vi "Lockin-4461 -Patrick -State -IV.vi"(11 "Channels: AO":T8={"AO amp (V)"=[1.0, 0.0, 0.0, 0.0, 0.0, 0.0, 0.0, 0.0], "AO DC (V)"=[0.0, 0.0, 0.0, 0.0, 0.0, 0.0, 0.0, 0.0], "AO f (Hz)"=[0.4, 0.4, 0.4, 0.4, 0.4, 0.4, 0.4, 0.4], "AO phi (deg)"=[0.0, 0.0, 0.0, 0.0, 0.0, 0.0, 0.0, 0.0], "function"=[enum."Triangle Wave", enum."Sine Wave", enum."Sine Wave", enum."Sine Wave", enum."Sine Wave", enum."Sine Wave", enum."Sine Wave", enum."Sine Wave"]} {"AO f (Hz)" min=0.001 max=1000.0; "AO DC (V)" format="%#_6p"; "AO amp (V)" format="%#_6p"}) -> ()   [LabVIEW 2013]
uses:
  <vilib>/Analysis/4window.llb/windowTd.ctl
  <vilib>/measure/maspectr.llb/Power Spectrum and PSD Export Mode.ctl
  <vilib>/Utility/error.llb/DialogType.ctl
  <vilib>/Analysis/baseanly.llb/Mean (DBL).vi
  <vilib>/Analysis/2dsp.llb/Decimate (single shot).vi
  <vilib>/Analysis/2dsp.llb/Decimate (single shot, DBL).vi
  <userlib>/_OpenG.lib/array/array.llb/Empty 1D Array (Variant)__ogtk.vi
  <userlib>/_OpenG.lib/array/array.llb/Empty 1D Array (DBL)__ogtk.vi
  <vilib>/measure/maspectr.llb/FFT Power Spectrum and PSD for N Chan.vi
  <vilib>/Waveform/WDTOps.llb/WDT Waveform to XY Pairs DBL.vi
  <vilib>/measure/NI_MAPro.lvlib
  <vilib>/Analysis/NI_AALBase.lvlib
  <vilib>/platform/TimedLoop/XDataNode/XDataNode.xnode
  <vilib>/Platform/TimedLoop/XDataNode/nitl_modes.ctl
  <vilib>/Platform/TimedLoop/XDataNode/XDNodeRunTimeDep.lvlib
  <vilib>/Platform/TimedLoop/XDataNode/wakeup.ctl
  <vilib>/Platform/TimedLoop/XDataNode/timing_clust.ctl
  <vilib>/Analysis/NI_AALPro.lvlib
panel:
  in  "save interval (s)":dbl=300.0
  out "save time":timestamp
  out "Error":bool
  out "Results\n(X, Y, R, Theta, mean)":dbl[][](array[numeric])=[[0.8094339767492822, -0.005512419987470585, 0.8094527469162581, -0.3901905858084899, -6.0129843950271606e-05], [-1.260821172105524e-07, 2.7497299313388556e-07, 3.0250098716087416e-07, 114.63266099744331, 0.0001555195415019989], [7.489149035008232e-07, 4.842270951726359e-07, 8.918236442172725e-07, 32.88556061807632, 8.126195073127747e-05], [-1.8506084817561703e-07, 1.6463385705296426e-07, 2.476930043735887e-07, 138.34306439782742, 0.0027563392603397368], [-4.6280871026111895e-07, 4.8028636431280393e-08, 4.652941566482524e-07, 174.07525665627907, 0.002910439200401306], [-4.1354357574928766e-07, 2.831131466682128e-07, 5.011699740206747e-07, 145.60434384741927, 0.0028921316146850585], [0.8094339767492822, -0.005512419987470585, 0.8094527469162581, -0.3901905858084899, 0.0], [-1.260821172105524e-07, 2.7497299313388556e-07, 3.0250098716087416e-07, 114.63266099744331, 0.0], [7.489149035008232e-07, 4.842270951726359e-07, 8.918236442172725e-07, 32.88556061807632, 0.0], [-1.8506084817561703e-07, 1.6463385705296426e-07, 2.476930043735887e-07, 138.34306439782742, 0.0], [-4.6280871026111895e-07, 4.8028636431280393e-08, 4.652941566482524e-07, 174.07525665627907, 0.0], [-4.1354357574928766e-07, 2.831131466682128e-07, 5.011699740206747e-07, 145.60434384741927, 0.0]] format="%#_3p"
  out "current time":timestamp=timestamp(3547741041.3268714 s since 1904-01-01)
  in  "Channel":dbl min=0.0 max=7.0 step=1.0
  in  "Display":enum16{"X and Y", "R and Theta"}(ring)
  out "Y or Theta":dbl=-0.005512419987470585 caption="Y or Theta: Current (A) or Voltage (V)" format="%.3p"
  out "X or R":dbl=0.8094339767492822 caption="X or R: Current (A) or Voltage (V)" format="%#.3p"
  in  "Save Data":bool
  in  "RESET":bool
  in  "EXIT":bool
  in  "path":path=path "C:/Data/lockin"
  in  "Notes":string
  in  "mean":dbl[](array[numeric])=[-6.0129843950271606e-05, 0.0001555195415019989, 8.126195073127747e-05, 0.0027563392603397368, 0.002910439200401306, 0.0028921316146850585]
  in  "Tab Control 2":T1(tab)
  in  "Output signals?":bool
  out "Signals Graph":waveform(dbl)[](graph)=[{"t0"=timestamp(3547741038.80007 s since 1904-01-01), "dt"=0.0002499999997785377, "Y"=array[10000 elements], "attributes"=variant("NI_ChannelName"=variant(string "PXI1Slot2/ai0"), "NI_UnitDescription"=variant(string "Volts"))}, {"t0"=timestamp(3547741038.80007 s since 1904-01-01), "dt"=0.0002499999997785377, "Y"=array[10000 elements], "attributes"=variant("NI_ChannelName"=variant(string "PXI1Slot2/ai1"), "NI_UnitDescription"=variant(string "Volts"))}, {"t0"=timestamp(3547741038.800245 s since 1904-01-01), "dt"=0.0002499999997785377, "Y"=array[10000 elements], "attributes"=variant("NI_ChannelName"=variant(string "PXI1Slot3/ai0"), "NI_UnitDescription"=variant(string "Volts"))}, {"t0"=timestamp(3547741038.800245 s since 1904-01-01), "dt"=0.0002499999997785377, "Y"=array[10000 elements], "attributes"=variant("NI_ChannelName"=variant(string "PXI1Slot3/ai1"), "NI_UnitDescription"=variant(string "Volts"))}, {"t0"=timestamp(3547741038.800295 s since 1904-01-01), "dt"=0.0002499999997785377, "Y"=array[10000 elements], "attributes"=variant("NI_ChannelName"=variant(string "PXI1Slot5/ai0"), "NI_UnitDescription"=variant(string "Volts"))}, {"t0"=timestamp(3547741038.800295 s since 1904-01-01), "dt"=0.0002499999997785377, "Y"=array[10000 elements], "attributes"=variant("NI_ChannelName"=variant(string "PXI1Slot5/ai1"), "NI_UnitDescription"=variant(string "Volts"))}]
  out "Reference Graph":waveform(dbl)[](graph)=[{"t0"=timestamp(3547741038.7997265 s since 1904-01-01), "dt"=0.00025, "Y"=array[10000 elements]}, {"t0"=timestamp(3547741038.7997265 s since 1904-01-01), "dt"=0.00025, "Y"=array[10000 elements]}, {"t0"=timestamp(3547741038.7997265 s since 1904-01-01), "dt"=0.00025, "Y"=array[10000 elements]}, {"t0"=timestamp(3547741038.7997265 s since 1904-01-01), "dt"=0.00025, "Y"=array[10000 elements]}, {"t0"=timestamp(3547741038.7997265 s since 1904-01-01), "dt"=0.00025, "Y"=array[10000 elements]}, {"t0"=timestamp(3547741038.7997265 s since 1904-01-01), "dt"=0.00025, "Y"=array[10000 elements]}, {"t0"=timestamp(3547741038.7997265 s since 1904-01-01), "dt"=0.00025, "Y"=array[10000 elements]}, {"t0"=timestamp(3547741038.7997265 s since 1904-01-01), "dt"=0.00025, "Y"=array[10000 elements]}]
  in  "decimate graph":i32=10
  in  "Display n?":bool
  out "Gauge":dbl(knob)=21.0 scale=0.0..60.0
  out "Display X (or R)":waveform(dbl)[](graph)=[{"t0"=timestamp(3547741038.80007 s since 1904-01-01), "dt"=1.0, "Y"=[0.8094339767492822]}, {"t0"=timestamp(3547741038.80007 s since 1904-01-01), "dt"=1.0, "Y"=[-1.260821172105524e-07]}, {"t0"=timestamp(3547741038.80007 s since 1904-01-01), "dt"=1.0, "Y"=[7.489149035008232e-07]}, {"t0"=timestamp(3547741038.80007 s since 1904-01-01), "dt"=1.0, "Y"=[-1.8506084817561703e-07]}, {"t0"=timestamp(3547741038.80007 s since 1904-01-01), "dt"=1.0, "Y"=[-4.6280871026111895e-07]}, {"t0"=timestamp(3547741038.80007 s since 1904-01-01), "dt"=1.0, "Y"=[-4.1354357574928766e-07]}, {"t0"=timestamp(3547741038.80007 s since 1904-01-01), "dt"=1.0, "Y"=[0.8094339767492822]}, {"t0"=timestamp(3547741038.80007 s since 1904-01-01), "dt"=1.0, "Y"=[-1.260821172105524e-07]}, {"t0"=timestamp(3547741038.80007 s since 1904-01-01), "dt"=1.0, "Y"=[7.489149035008232e-07]}, {"t0"=timestamp(3547741038.80007 s since 1904-01-01), "dt"=1.0, "Y"=[-1.8506084817561703e-07]}, {"t0"=timestamp(3547741038.80007 s since 1904-01-01), "dt"=1.0, "Y"=[-4.6280871026111895e-07]}, {"t0"=timestamp(3547741038.80007 s since 1904-01-01), "dt"=1.0, "Y"=[-4.1354357574928766e-07]}]
  out "Display Y (or Theta)":waveform(dbl)[](graph)=[{"t0"=timestamp(3547741038.80007 s since 1904-01-01), "dt"=1.0, "Y"=[-0.005512419987470585]}, {"t0"=timestamp(3547741038.80007 s since 1904-01-01), "dt"=1.0, "Y"=[2.7497299313388556e-07]}, {"t0"=timestamp(3547741038.80007 s since 1904-01-01), "dt"=1.0, "Y"=[4.842270951726359e-07]}, {"t0"=timestamp(3547741038.80007 s since 1904-01-01), "dt"=1.0, "Y"=[1.6463385705296426e-07]}, {"t0"=timestamp(3547741038.80007 s since 1904-01-01), "dt"=1.0, "Y"=[4.8028636431280393e-08]}, {"t0"=timestamp(3547741038.80007 s since 1904-01-01), "dt"=1.0, "Y"=[2.831131466682128e-07]}, {"t0"=timestamp(3547741038.80007 s since 1904-01-01), "dt"=1.0, "Y"=[-0.005512419987470585]}, {"t0"=timestamp(3547741038.80007 s since 1904-01-01), "dt"=1.0, "Y"=[2.7497299313388556e-07]}, {"t0"=timestamp(3547741038.80007 s since 1904-01-01), "dt"=1.0, "Y"=[4.842270951726359e-07]}, {"t0"=timestamp(3547741038.80007 s since 1904-01-01), "dt"=1.0, "Y"=[1.6463385705296426e-07]}, {"t0"=timestamp(3547741038.80007 s since 1904-01-01), "dt"=1.0, "Y"=[4.8028636431280393e-08]}, {"t0"=timestamp(3547741038.80007 s since 1904-01-01), "dt"=1.0, "Y"=[2.831131466682128e-07]}]
  out "XY Graph":cluster{dbl[], dbl[]}[](graph)=[{[0.0, 0.8094339767492822], [0.0, -0.005512419987470585]}, {[0.0, -1.260821172105524e-07], [0.0, 2.7497299313388556e-07]}, {[0.0, 7.489149035008232e-07], [0.0, 4.842270951726359e-07]}, {[0.0, -1.8506084817561703e-07], [0.0, 1.6463385705296426e-07]}, {[0.0, -4.6280871026111895e-07], [0.0, 4.8028636431280393e-08]}, {[0.0, -4.1354357574928766e-07], [0.0, 2.831131466682128e-07]}, {[0.0, 0.8094339767492822], [0.0, -0.005512419987470585]}, {[0.0, -1.260821172105524e-07], [0.0, 2.7497299313388556e-07]}, {[0.0, 7.489149035008232e-07], [0.0, 4.842270951726359e-07]}, {[0.0, -1.8506084817561703e-07], [0.0, 1.6463385705296426e-07]}, {[0.0, -4.6280871026111895e-07], [0.0, 4.8028636431280393e-08]}, {[0.0, -4.1354357574928766e-07], [0.0, 2.831131466682128e-07]}]
  out "PS Chart":dbl[][](graph)=[[-1411.497616925462, -1404.3790029743438, -1413.0961920610762, -1418.6418791322994, -1413.136726104145, -1413.4151534226191, -1417.9246313001065, -1424.6072395567076]]
  out "PS dB":cluster{"f0":dbl, "df":dbl, "magnitude":dbl[]}[](graph)
  in  "window":T2=1 items=["Rectangle"=0, "Hanning"=1, "Hamming"=2, "Blackman-Harris"=3, "Exact Blackman"=4, "Blackman"=5, "Flat Top"=6, "4 Term B-Harris "=7, "7 Term B-Harris"=8, "Low Sidelobe"=9, "Blackman Nuttall"=11, "Triangle"=30, "Bartlett-Hanning"=31, "Bohman"=32, "Parzen"=33, "Welch"=34, "Kaiser"=60, "Dolph-Chebyshev"=61, "Gaussian"=62]
  in  "averaging parameters":T3={"averaging mode"=enum."RMS averaging", "weighting mode"=enum."Exponential", "number of averages"=10} {"number of averages" min=1}
  in  "restart averaging (F)":bool
  in  "export mode":T4 items=["Power Spectrum", "Power Spectral Density"]
  in  "window parameter":dbl=nan
  out "averages\ncompleted":dbl=8319.0
  out "averaging done":bool=TRUE
  in  "Tab Control":T5(tab)=enum."AO/Lockin Setup"
  in  "decimating factor":i32=1
  in  "AI Buffer Size (S)":i32=100
  out "dt":dbl=2.5e-05 format="%#_6p"
  in  "AO Configuration":T6(array[cluster])=[{"Output physical channels"="PXI1Slot2/ao0:1", "AO. Max"=1.0, "AO.Min"=-1.0}, {"Output physical channels"="PXI1Slot3/ao0:1", "AO. Max"=1.0, "AO.Min"=-1.0}, {"Output physical channels"="PXI1Slot5/ao0:1", "AO. Max"=1.0, "AO.Min"=-1.0}]
  in  "AI Configuration":T7(array[cluster])=[{"AI.Coupling"=10050, "AI.Max"=1.0, "AI.Min"=-1.0, "Input physical channels"="PXI1Slot2/ai0:1"}, {"AI.Coupling"=10050, "AI.Max"=1.0, "AI.Min"=-1.0, "Input physical channels"="PXI1Slot3/ai0:1"}, {"AI.Coupling"=10050, "AI.Max"=1.0, "AI.Min"=-1.0, "Input physical channels"="PXI1Slot5/ai0:1"}] {"AI.Coupling" items=["AC"=10045, "DC"=10050, "GND"=10066]}
  out "error":errorcluster
  in  "IV curves?":bool=TRUE
  in  "measure offset":bool
  in  "reset signal":bool
  in  "all  f same?":bool
  in  "reset REF phi to zero":bool
  in  "zero offset":bool
  in  "LP cutoff (Hz)":dbl=10.0
  in  "LP prefilter":bool
  in  "60 Hz prefilter":bool
  in  "Wait on Trigger":bool
  in  "Remote Mode":bool
  in  "Channels: Lockin":T9={"REF f (Hz)"=[0.4, 0.4], "REF phi (deg)"=[0.0, 0.0]} {"REF phi (deg)" format="%#_3g"}
  in  "simulate?":bool
  in  "order":i32=2
  in  "TC (s)":dbl=0.01 format="%#_6p"
  out "filter fC (Hz)":dbl=0.3183098861837907
  in  "autophase?\n(experimental)":bool
  in  "P":dbl=0.5 format="%.2f"
  in  "I":dbl=0.6 format="%.2f"
  in  "D":dbl=0.019999999999999997 format="%.2f"
  out "time since trigger":dbl
  in  "auto block size":bool=TRUE
  in  "x":dbl=100000.0 format="%#_13g"
  in  "sampling info":cluster{"Fs":i32, "#s":i32}={"Fs"=40000, "#s"=100000}
  in  "offsets":dbl[](array[numeric])=[0.0, 0.0, 0.0, 0.0, 0.0, 0.0, 0.0, 0.0] format="%#.2p"
  in  "Gain":dbl[](array[numeric])=[1.0, 1.0, 1.0, 1.0, 1.0, 1.0, 1.0, 1.0]
  out "phase log":dbl[](array[numeric])=[12.0, 12.0, 12.0, 12.0, 12.0, 12.0, 12.0, 12.0] format="%.1f"
  # "´"
  # "Multichannel Lockin v2016/06/02 IV"
  # "this is disabled!"
  # "plot 0    = AI0 f0\nplot 1    = Ai1 f0\n...\nplot N-1  = AIN f0\n\nplot N    = AI0 f1\nplot N+1  = AI1 f1\n..."
  # "sampling"
  # "prefilters"
  # "Make fs x*f0"
  # "lockin filter"
  # "autophase"
  # "0"
  # "1"
  # "2"
  # "3"
  # "4"
  # "5"
  # "6"
  # "7"
  # "Random Thoughts\n1. change the path in the yellow box below where you want to save the signal traces for diagnostics\n(G:\\ on CustardPie, H:\\ on WindySea)\n2. Change the AI and AO limits on the DAQ Settings tab\n\nPlease email p.irvin@levylab.org with questions or suggestions. Thanks."
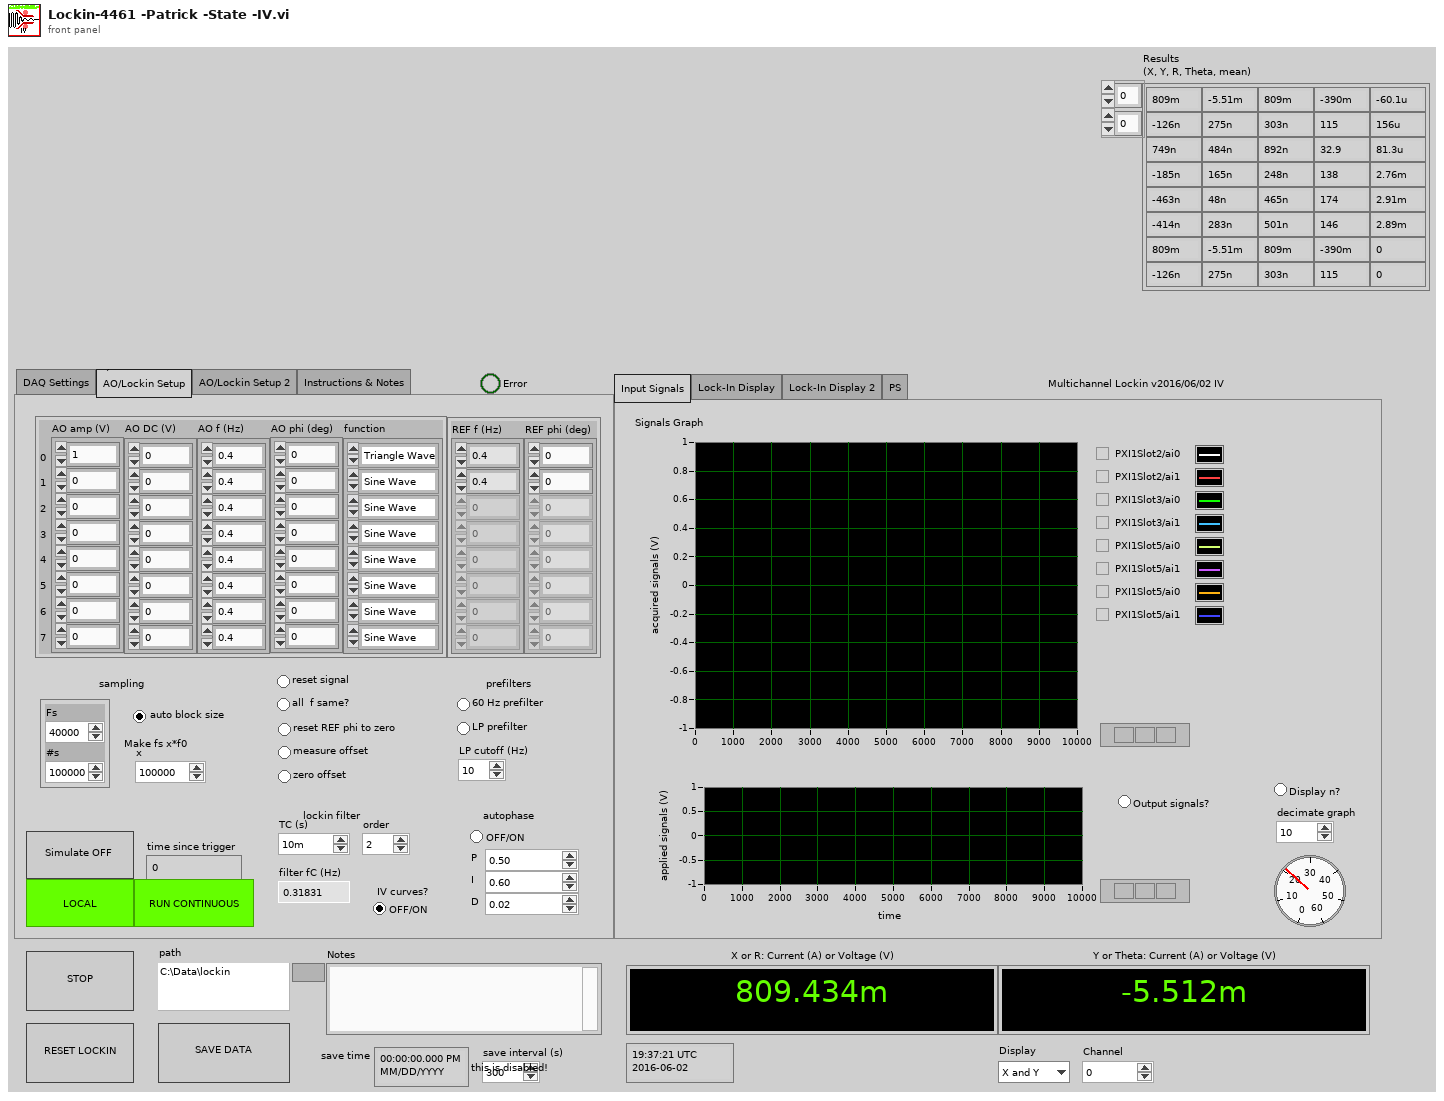
[diagram p1: front panel]
types:
  T1 = enum32{"Input Signals", "Lock-In Display", "Lock-In Display 2", "PS"}
  T2 = typedef "NI_AALPro.lvlib/windowTd.ctl" = u32
  T3 = cluster{"averaging mode":enum16{"No averaging", "Vector averaging", "RMS averaging", "Peak hold"}, "weighting mode":enum16{"Linear", "Exponential"}, "number of averages":u32}
  T4 = typedef "NI_MAPro.lvlib/Power Spectrum and PSD Export Mode.ctl" = u16
  T5 = enum32{"DAQ Settings", "AO/Lockin Setup", "AO/Lockin Setup 2", "Instructions & Notes"}
  T6 = cluster{"Output physical channels":tag, "AO. Max":dbl, "AO.Min":dbl}[]
  T7 = cluster{"AI.Coupling":i32, "AI.Max":dbl, "AI.Min":dbl, "Input physical channels":tag}[]
  T8 = cluster{"AO amp (V)":dbl[], "AO DC (V)":dbl[], "AO f (Hz)":dbl[], "AO phi (deg)":dbl[], "function":enum16{"Sine Wave", "Triangle Wave", "Square Wave", "Sawtooth Wave"}[]}
  T9 = cluster{"REF f (Hz)":dbl[], "REF phi (deg)":dbl[]}
  T10 = typedef "XDNodeRunTimeDep.lvlib/timing_clust.ctl" = cluster{"Expected End [f-1]":u64, "Actual End [f-1]":u64, "Finished Late? [f-1]":bool, "Expected End [i-1]":u64, "Actual End [i-1]":u64, "Finished Late? [i-1]":bool, "Expected Start [i]":u64, "Actual Start [i]":u64, "Expected Start [f]":u64, "Actual Start [f]":u64, "Source Name":string, "Structure Name":string, "Period":i64, "Deadline":i64, "Offset":i64, "Start":i64, "Priority":i32, "Timeout":i32, "Mode":T11, "Wakeup Reason":T12, "Error":errorcluster, "Source Type":string, "Secondary Source Type":string, "Global End Time":u64, "Global Start Time":u64, "Frame Duration":u64, "Iteration Duration":u64, "Assigned CPU":i32, "I/O Scan Engine Mode":u32}
  T11 = typedef "XDNodeRunTimeDep.lvlib/nitl_modes.ctl" = enum32{"No Change", "Process missed periods, maintain original phase", "Discard missed periods, maintain original phase", "Process missed periods, ignore original phase", "Discard missed periods, ignore original phase"}
  T12 = typedef "XDNodeRunTimeDep.lvlib/wakeup.ctl" = enum32{"Normal", "Aborted", "Asynchronous wakeup", "Timing source error", "Timed loop error", "Timeout"}
  T13 = enum32{"invalid app kind", "Development System", "Run Time System", "Student Edition", "Embedded LabVIEW", "Evaluation", "Custom"}
  T14 = enum32{"Invalid", "Standard", "Closed", "Hidden", "Minimized", "Maximized"}
  T15 = enum32{"Input Signals", "Lock-In Display", "Lock-In Display 2", "PS", "FFT"}
  T16 = cluster{"Core":cluster{"Current VI Reference":refnum<vi>, "Close Panel on Exit?":bool}, "Error":bool, "Your string data":string, "AI task":refnum<k21>[], "AO task":refnum<k21>[], "Input Signals":waveform(dbl)[], "Ouput Signals":waveform(dbl)[], "REF":waveform(dbl)[], "sampling info":cluster{"Fs":dbl, "#s":dbl}}
  T17 = typedef "DialogType.ctl" = u16
  T18 = cluster{"Current VI Reference":refnum<vi>, "Close Panel on Exit?":bool}
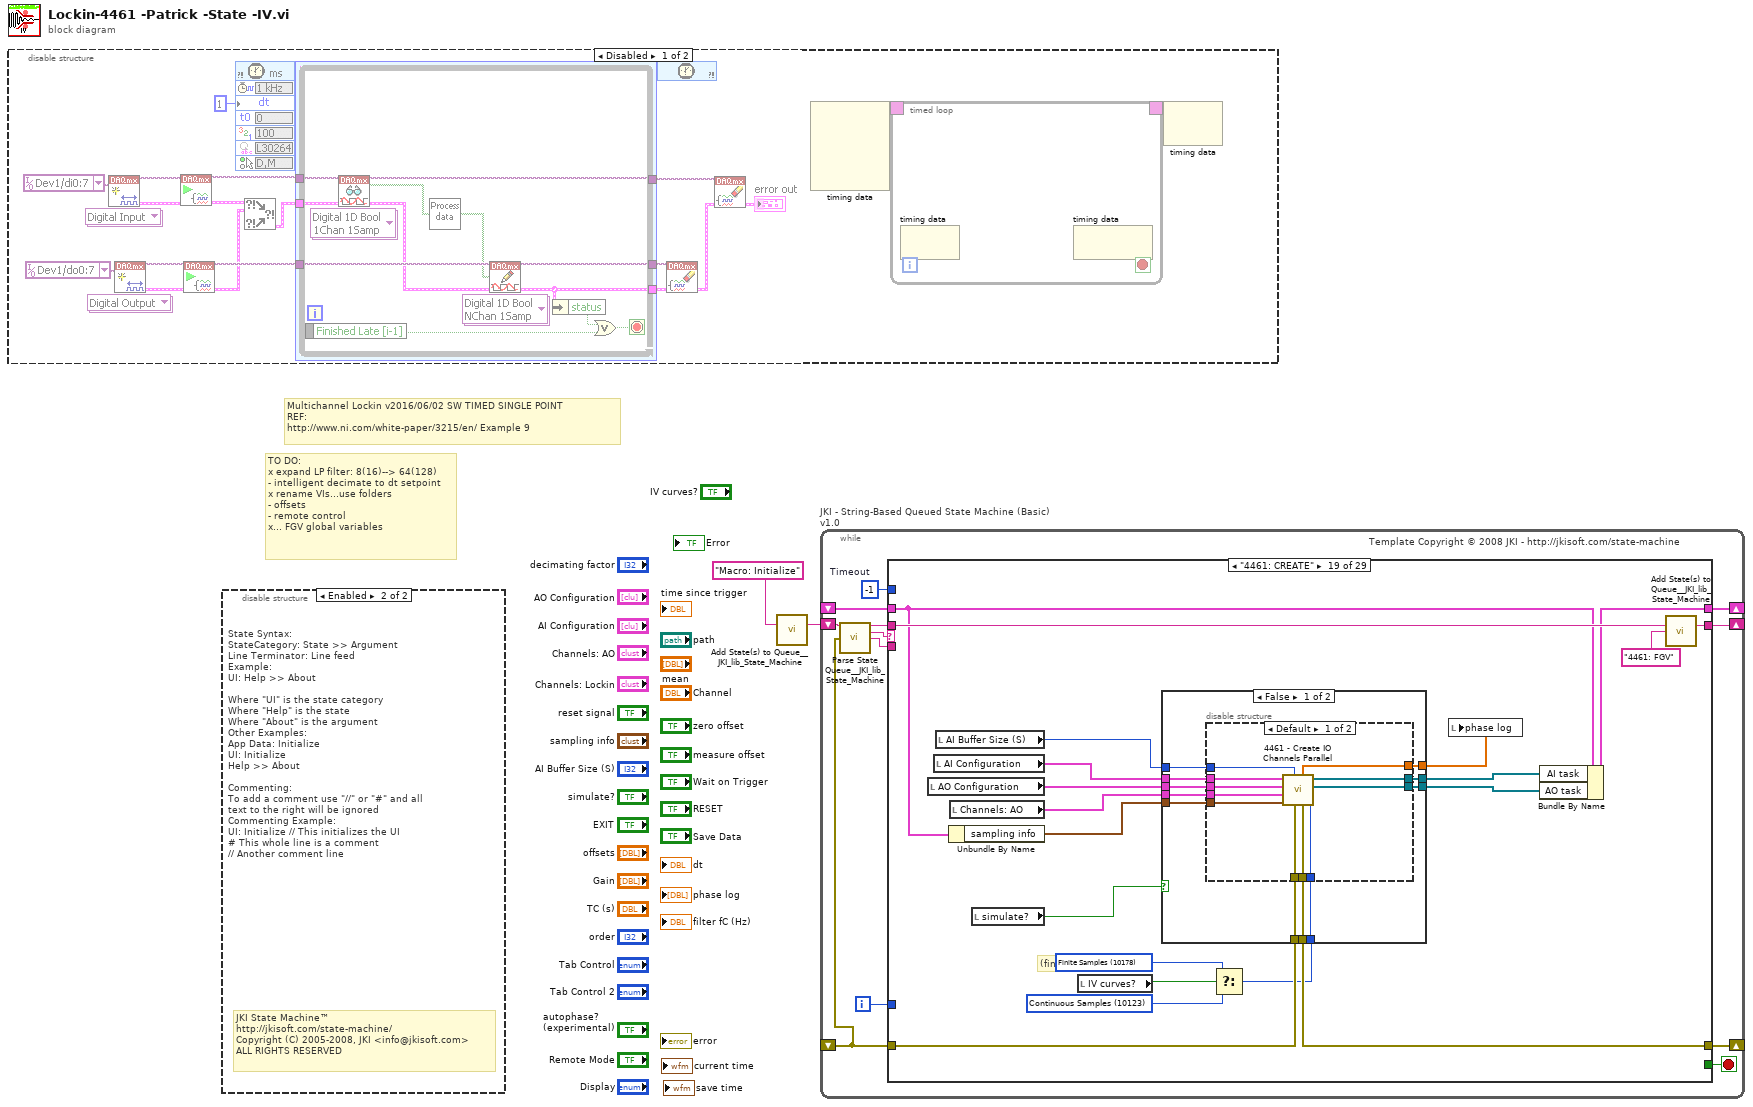
[diagram p0: block diagram]
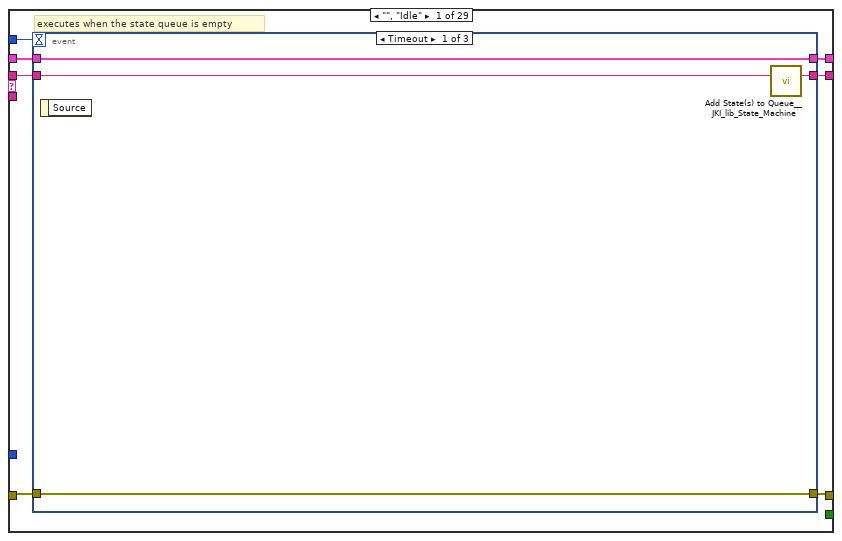
[diagram p4: hidden frame]
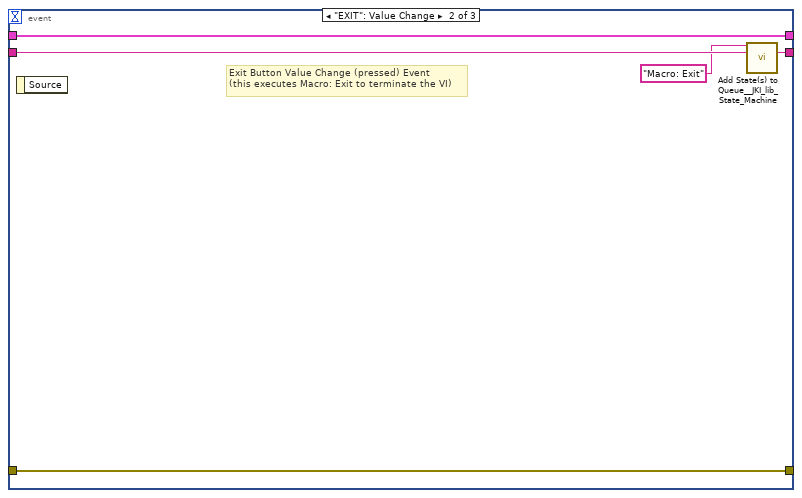
[diagram p5: hidden frame]
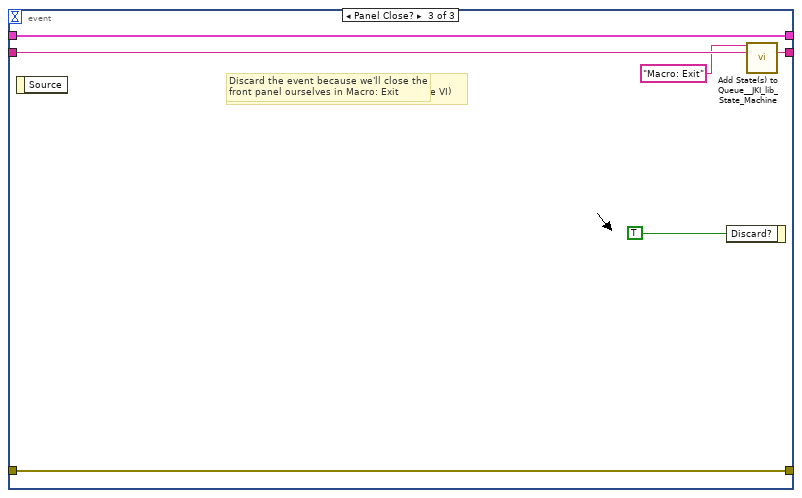
[diagram p6: hidden frame]
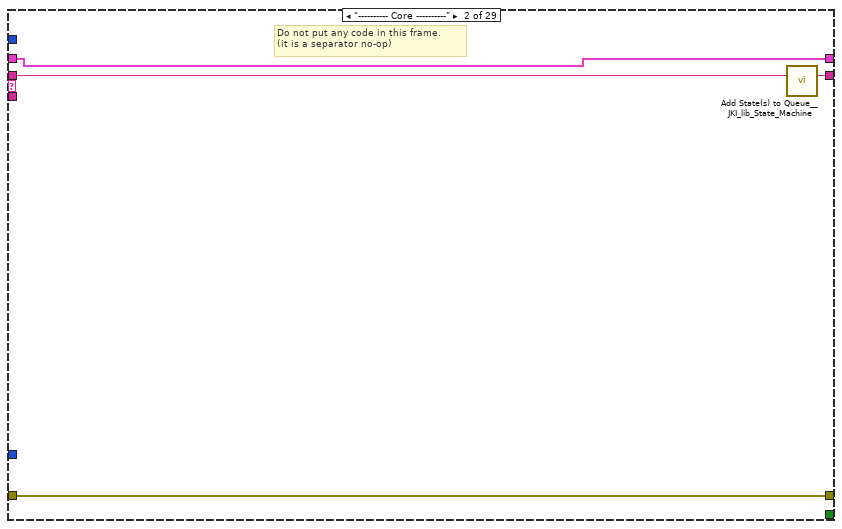
[diagram p7: hidden frame]
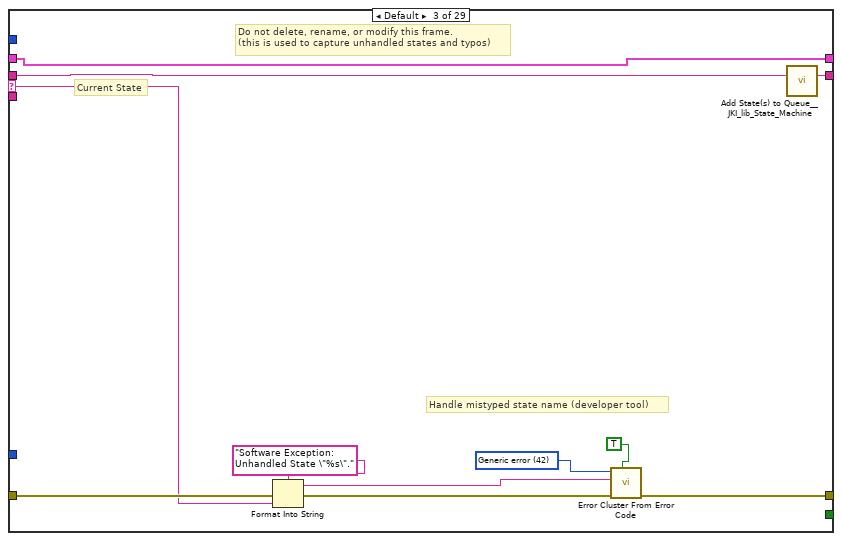
[diagram p8: hidden frame]
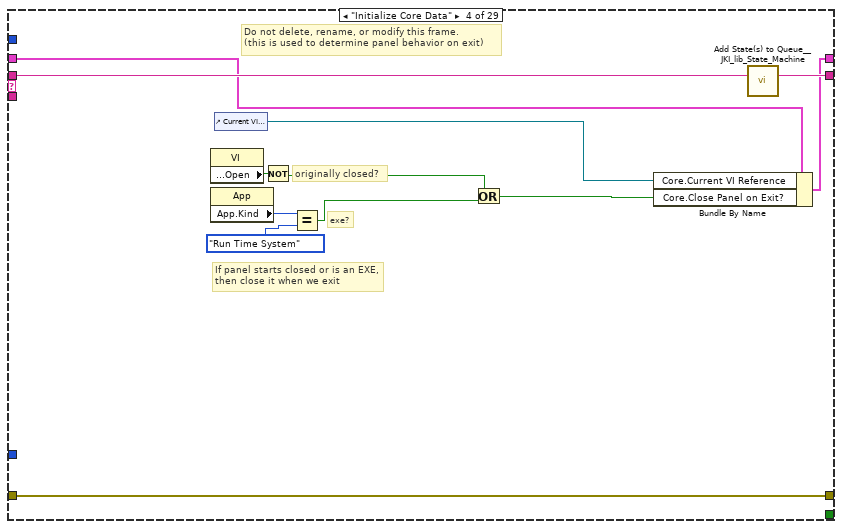
[diagram p9: hidden frame]
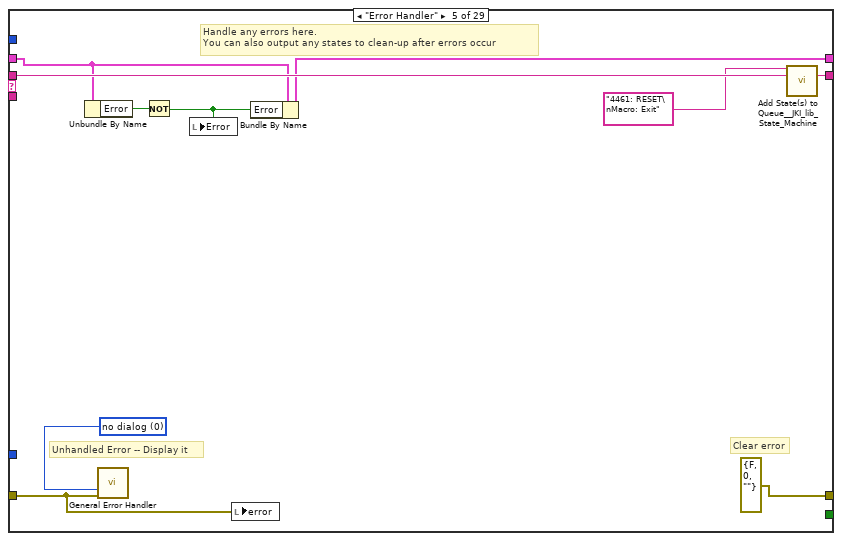
[diagram p10: hidden frame]
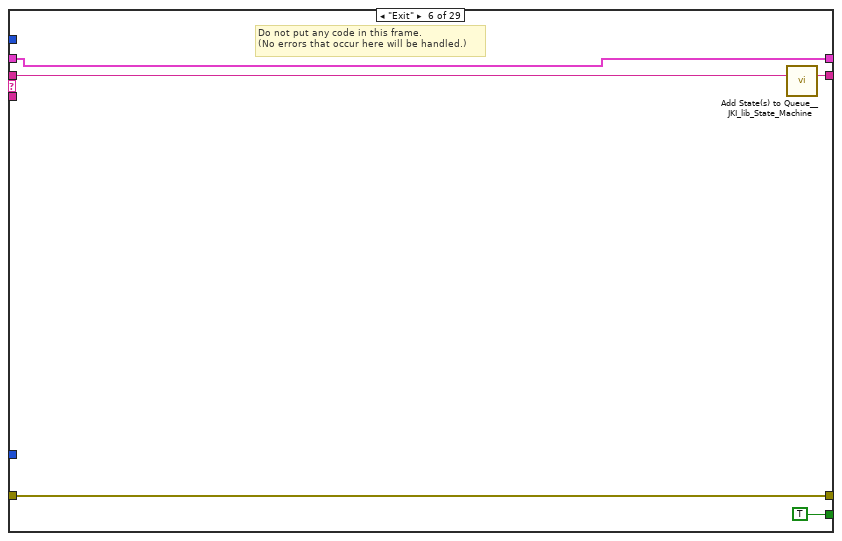
[diagram p11: hidden frame]
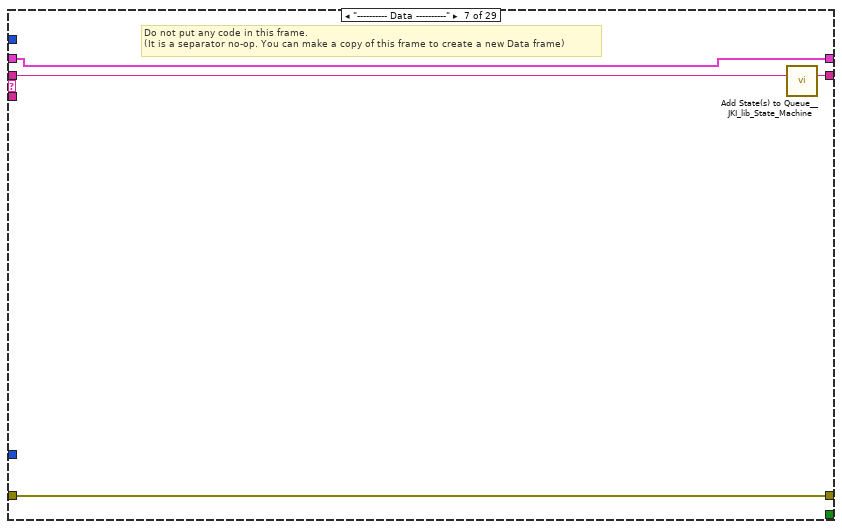
[diagram p12: hidden frame]
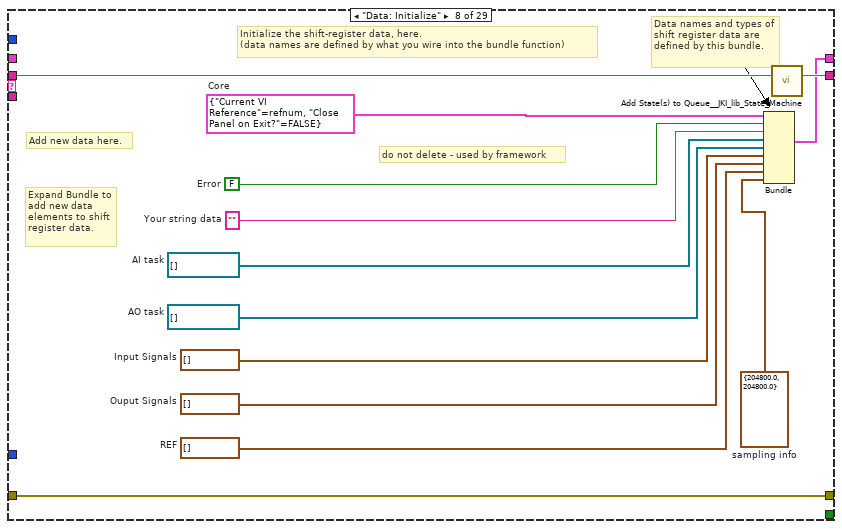
[diagram p13: hidden frame]
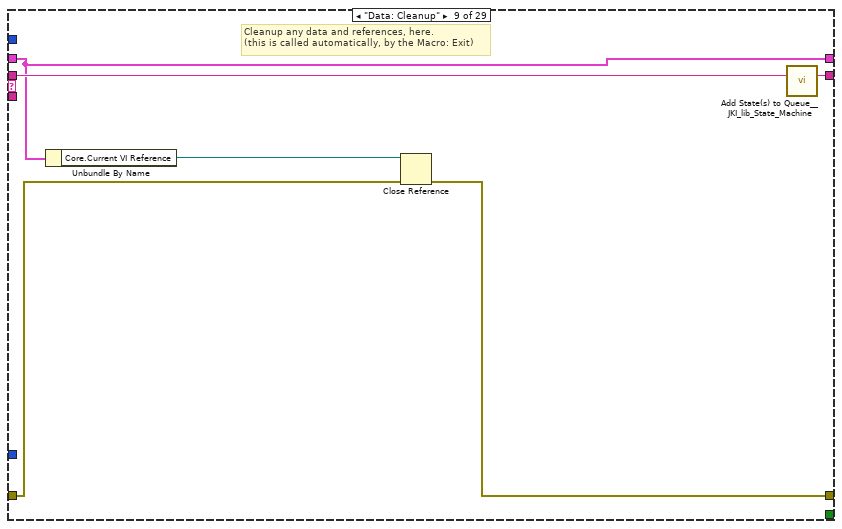
[diagram p14: hidden frame]
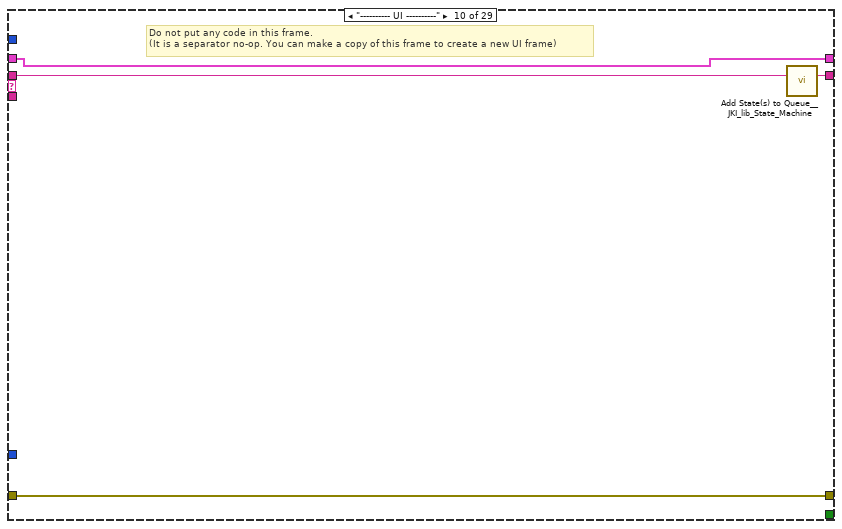
[diagram p15: hidden frame]
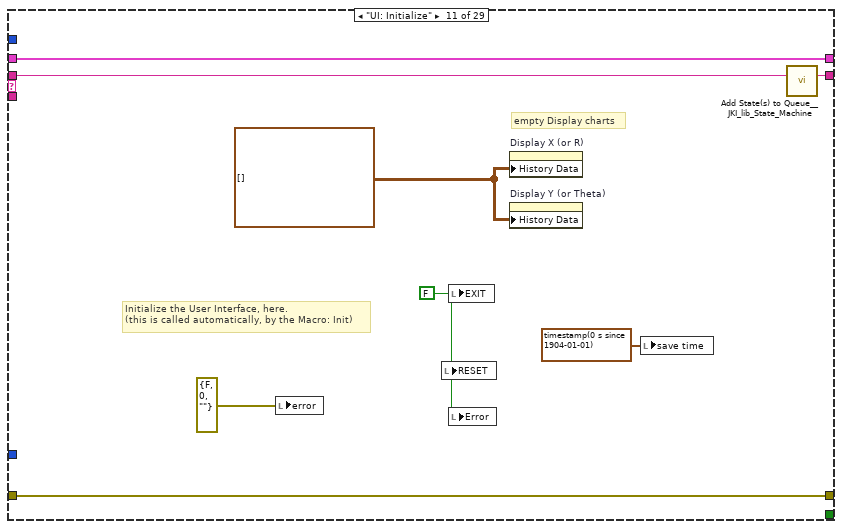
[diagram p16: hidden frame]
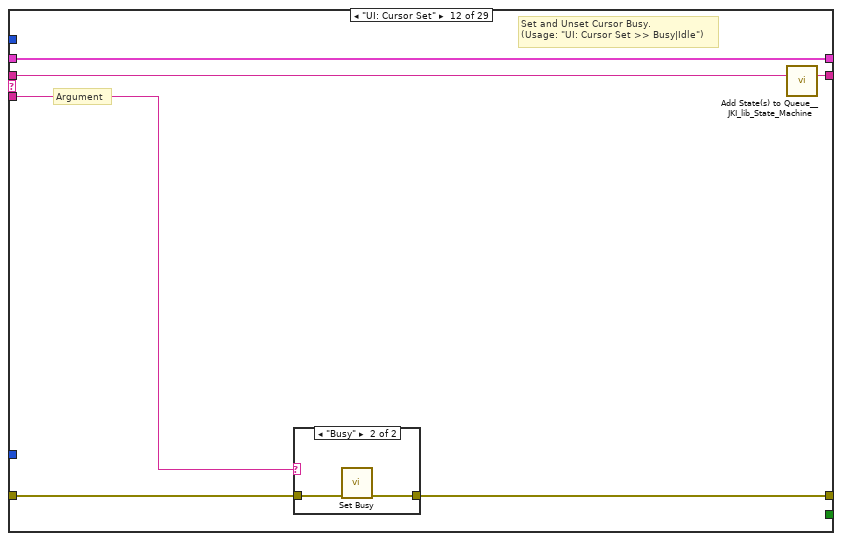
[diagram p17: hidden frame]
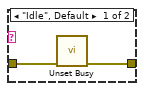
[diagram p18: hidden frame]
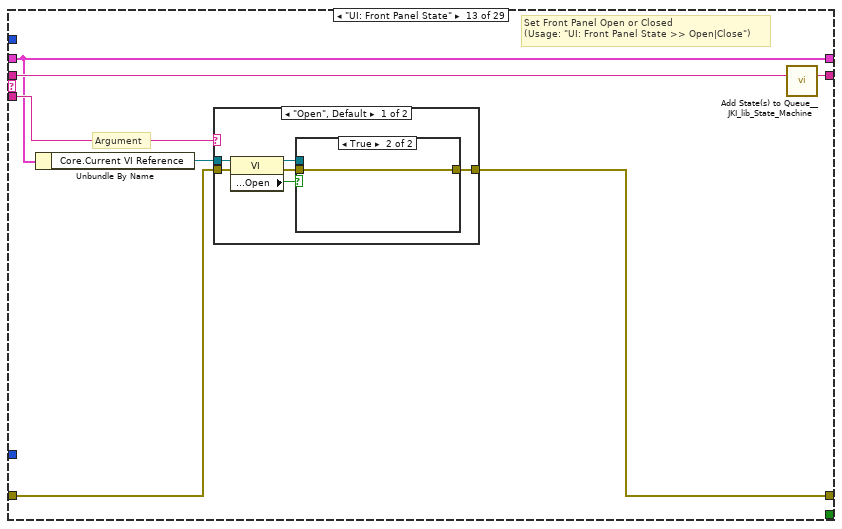
[diagram p19: hidden frame]
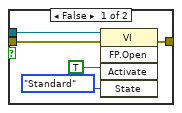
[diagram p20: hidden frame]
diagram:
  # "Multichannel Lockin v2016/06/02 SW TIMED SINGLE POINT\nREF:\nhttp://www.ni.com/white-paper/3215/en/ Example 9"
  # "TO DO:\nx expand LP filter: 8(16)--> 64(128)\n- intelligent decimate to dt setpoint\nx rename VIs...use folders\n- offsets\n- remote control\nx... FGV global variables"
  n1 = disable-structure shown="Disabled" {
    frame Disabled {
      n2 = node-c288() -> (w4:T10)  [unwired: 4 in]
      n3 = timed-loop {
        timing: w4 -> [_]
        timing-out: [_] -> w3
        stop <- _ stop-if-true
        n4 = node-c288() -> ()  [unwired: 1 in, 1 out]
        n5 = node-c288() -> ()  [unwired: 1 in, 1 out]
      }
      n6 = node-c288(w3) -> ()  [unwired: 1 out]
    }
    frame Enabled {
    }
  }
  n7 = disable-structure shown="Enabled" {
    frame Disabled {
    }
    frame Enabled {
      # "JKI State Machine™\nhttp://jkisoft.com/state-machine/\nCopyright (C) 2005-2008, JKI <info@jkisoft.com>\nALL RIGHTS RESERVED"
      # "State Syntax:\nStateCategory: State >> Argument\nLine Terminator: Line feed\nExample:\nUI: Help >> About\n\nWhere \"UI\" is the state category\nWhere \"Help\" is the state\nWhere \"About\" is the argument\nOther Examples:\nApp Data: Initialize\nUI: Initialize\nHelp >> About\n\nCommenting:\nTo add a comment use \"//\" or \"#\" and all text to the right will be ignored\nCommenting Example:\nUI: Initialize // This initializes the UI\n# This whole line is a comment\n// Another comment line"
    }
  }
  n8 = call <vilib>:"Add State(s) to Queue__JKI_lib_State_Machine.vi"("State(s) in (\"\")"="Macro: Initialize") -> ("States Out"=w2:string)  [unwired: 14 in]
  n9 = while "JKI - String-Based Queued State Machine (Basic) v1.0" {
    shift-right: [w14] -> _
    shift-left: _ -> [w13]
    shift-right: [w17] -> _
    shift-left: _ -> [w11]
    shift-right: [w16] -> _
    shift-left: w2 -> [w18]
    i -> [w9]
    stop <- w15 stop-if-true
    w12 = -1  # Timeout
    # "Template Copyright © 2008 JKI - http://jkisoft.com/state-machine"
    n10 = call <vilib>:"Parse State Queue__JKI_lib_State_Machine.vi"("State Queue"=w18, "Error In (no error)"=w11) -> ("Remaining States"=w10:string, "Current State"=w20:string, "Arguments"=w19:string)  [unwired: 11 in]
    n11 = case shown="\"4461: CREATE\"" w20 {
      selector: w20 -> [_ _ w47 _ _ _ _ _ _ _ _ _ _ _ _ _ _ _ _ _ _ _ _ _ _ _ _ _ _]
      tunnel: w19 -> [_ _ _ _ _ _ _ _ _ _ _ w121 w132 _ _ _ _ _ _ _ _ _ _ _ _ _ _ _ _]
      tunnel: w13 -> [w25 w43 w49 w60 w72 w82 w85 _ w102 w108 w116 w120 w131 w159 w163 w168 w179 w187 w234 w301 w325 w366 w425 w446 w562 w596 w635 w670 w710]
      tunnel: [w24 w44 w53 w66 errorcluster {"status"=FALSE, "code"=0, "source"=""} ("error out") w81 w86 w98 w103 w109 w114 w122 w130 w160 w165 w176 w180 w197 w236 w294 w335 w380 w414 w443 w564 w590 w625 w664 w708] -> w17
      tunnel: w11 -> [w23 w44 w52 w66 w74 w81 w86 w98 w104 w109 w114 w123 w134 w160 w165 w176 w180 w193 w240 w290 w337 w383 w414 w444 w564 w592 w624 w665 w709]
      tunnel: [w26 w45 w50 w68 w78 w83 w87 w100 w106 w110 w118 w124 w135 w161 w166 w177 w181 w208 w247 w300 w339 w391 w426 w442 w563 w597 w636 w666 w714] -> w16
      tunnel: [_ _ _ _ _ TRUE _ _ _ _ _ _ _ _ _ _ _ _ _ _ _ _ _ _ _ _ _ _ _] -> w15
      tunnel: [w22 w43 w49 w67 w71 w82 w85 w99 w102 w108 w116 w120 w131 w159 w163 w168 w179 w185 w242 w301 w338 w390 w425 w441 w562 w596 w635 w670 w710] -> w14
      tunnel: w12 -> [w21 _ _ _ _ _ _ _ _ _ _ _ _ _ _ _ _ _ _ _ _ _ _ _ _ _ _ _ _]
      tunnel: w10 -> [w27 w46 w51 w69 w79 w84 w88 w101 w107 w111 w119 w125 w136 w162 w167 w178 w182 w209 w248 w299 w340 w392 w427 w445 w565 w598 w637 w668 w714]
      tunnel: w9 -> [_ _ _ _ _ _ _ _ _ _ _ _ _ _ _ _ _ _ _ _ _ _ _ _ _ _ _ _ w713]
      frame "", "Idle" {
        # "executes when the state queue is empty"
        n12 = event shown="[0] Timeout" {
          selector: _ -> [_ _ _]
          dyn-events: _ -> [_ _ _]
          timeout: w21 -> [_ _ _]
          tunnel: w27 -> [w31 w36 w42]
          tunnel: [w30 w35 w41] -> w26
          tunnel: w25 -> [w28 w33 w39]
          tunnel: [w29 w34 w40] -> w24
          tunnel: w23 -> [w29 w34 w40]
          tunnel: [w28 w33 w39] -> w22
          event Timeout {
            n13 = event-data() -> ()  [unwired: 1 in, 1 out]
            n14 = call <vilib>:"Add State(s) to Queue__JKI_lib_State_Machine.vi"("State(s) in (\"\")"=w31) -> ("States Out"=w30:string)  [unwired: 14 in]
          }
          event "EXIT": Value Change {
            # "Exit Button Value Change (pressed) Event\n(this executes Macro: Exit to terminate the VI)"
            n15 = event-data() -> ()  [unwired: 1 in, 1 out]
            n16 = call <vilib>:"Add State(s) to Queue__JKI_lib_State_Machine.vi"("State(s) in Front (\"\")"="Macro: Exit", "State(s) in (\"\")"=w36) -> ("States Out"=w35:string)  [unwired: 13 in]
          }
          event Panel Close? {
            # "Discard the event because we'll close the front panel ourselves in Macro: Exit"
            # "Close Panel button (pressed) Event\n(this executes Macro: Exit to terminate the VI)"
            n17 = event-data() -> ()  [unwired: 1 in, 1 out]
            n18 = event-data("Discard?"=TRUE) -> ()  [unwired: 1 in, 1 out]
            n19 = call <vilib>:"Add State(s) to Queue__JKI_lib_State_Machine.vi"("State(s) in Front (\"\")"="Macro: Exit", "State(s) in (\"\")"=w42) -> ("States Out"=w41:string)  [unwired: 13 in]
          }
        }
      }
      frame "---------- Core ----------" {
        # "Do not put any code in this frame.\n(it is a separator no-op)"
        n20 = call <vilib>:"Add State(s) to Queue__JKI_lib_State_Machine.vi"("State(s) in (\"\")"=w46) -> ("States Out"=w45:string)  [unwired: 14 in]
      }
      frame Default {
        w56 = 42 items=["No error", "Argument error", "Memory is full", "Out of zone", "End of file", "File already open", "Generic file I/O error", "File not found", "File permission error", "Disk is full", "Duplicate path", "Too many files open", "System feature not enabled", "Resource file not found", "Cannot add resource", "Resource not found", "Image not found", "Image memory error", "Pen does not exist", "Config type invalid", "Config token not found", "Config parse error", "Config memory error", "Bad external code format", "Bad external code offset", "External code not present", "Null window", "Destroy window error", "Null menu", "Print aborted", "Bad print record", "Print driver error", "Windows error during printing", "Memory error during printing", "Print dialog error", "Generic print error", "Invalid device refnum", "Device not found", "Device parameter error", "Device unit error", "Cannot open device", "Device call aborted", "Generic error", "Cancelled by user", "Object ID too low", "Object ID too high", "Object not in heap", "Unknown heap", "Unknown object (invalid DefProc)", "Unknown object (DefProc not in table)", "Message out of range", "Invalid (null) method", "Unknown message", "Manager call not supported", "Bad address", "Network operation in progress", "Network operation timed out", "Connection is busy", "Network attribute not supported", "Network error", "Address in use", "System out of memory", "Connection aborted", "Connection refused", "Not connected", "Already connected", "Connection closed", "Initialization error (interapplication manager)", "Bad occurrence", "Wait on unbound occurrence handler", "Occurrence queue overflow", "Datalog type conflict", "Unused", "Unrecognized type (interapplication manager)", "Memory corrupt", "Failed to make temporary DLL", "Old CIN version", "Drag socket not found", "Failed to load drop-object", "Failed to register OLE object", "Failed to release OLE object", "Format specifier type mismatch", "Unknown format specifier", "Too few format specifiers", "Too many format specifiers", "Scan failed", "Newer CIN version", "Error converting to variant", "Runtime menu error", "Password tampered", "Variant attribute not found", "Incompatible variant data type", "Event data is not available", "Event Store is not present", "Occurrence is not found", "Event Queue is not created", "Event info is not available", "Refnum passed is NULL", "Error retrieving Class GUID", "Error retrieving CoClass GUID", "Error retrieving TypeLib GUID.", "Bad built application magic bytes.", "Specific driver is different from the specific driver associated with the Logical Name.", "There is no session opened to the class driver.", "Max Error", "MAX - Error with config objects", "MAX - Error loading configuration", "MAX - Group not supported"]
        # "Current State"
        # "Do not delete, rename, or modify this frame.\n(this is used to capture unhandled states and typos)"
        # "Handle mistyped state name (developer tool)"
        n21 = Format Into String(format string="Software Exception: Unhandled State \"%s\"." ("message"), error in=w52, w47) -> (resulting string=w55:string, error out=w54:errorcluster)  [unwired: 1 in]
        n22 = call <vilib>:"Error Cluster From Error Code.vi"("show call chain? (False)"=TRUE, "error in (no error)"=w54, "error message (\"\")"=w55, "error code (0)"=w56) -> ("error out"=w53:errorcluster)  [unwired: 5 in]
        n23 = call <vilib>:"Add State(s) to Queue__JKI_lib_State_Machine.vi"("State(s) in (\"\")"=w51) -> ("States Out"=w50:string)  [unwired: 14 in]
      }
      frame "Initialize Core Data" {
        # "Do not delete, rename, or modify this frame.\n(this is used to determine panel behavior on exit)"
        # "originally closed?"
        # "exe?"
        # "If panel starts closed or is an EXE, then close it when we exit"
        n24 = property class="VI"() -> ("Front Panel.Open"=w65:bool)  [unwired: 2 in, 2 out]
        n25 = property class="App"() -> ("App.Kind"=w64:T13)  [unwired: 2 in, 2 out]
        n26 = control-ref of="Current VI Reference"() -> (w58:refnum<vi>)
        n27 = Not(x=w65) -> (.not. x?=w62:bool)
        n28 = Equal?(x=w64, y=T13."Run Time System" ("Application:Kind")) -> (x = y?=w61:bool)
        n29 = Or(x=w62, y=w61) -> (x .or. y?=w59:bool)
        n30 = Bundle By Name(cluster=w60, "Core.Current VI Reference"=w58, "Core.Close Panel on Exit?"=w59) -> (w67:T16)
        n31 = call <vilib>:"Add State(s) to Queue__JKI_lib_State_Machine.vi"("State(s) in (\"\")"=w69) -> ("States Out"=w68:string)  [unwired: 14 in]
      }
      frame "Error Handler" {
        w75 = T17 0 items=["no dialog", "OK message", "continue or stop message", "OK message + warnings", "continue/stop + warnings"] ("type of dialog (OK msg:1)")
        # "Unhandled Error -- Display it"
        # "Handle any errors here.\nYou can also output any states to clean-up after errors occur"
        # "Clear error"
        n32 = Unbundle By Name(w72) -> ("Error"=w73:bool)
        n33 = call <vilib>:"General Error Handler.vi"("type of dialog (OK msg:1)"=w75, "error in (no error)"=w74) -> ()  [unwired: 9 in, 5 out]
        n34 = Not(x=w73) -> (.not. x?=w70:bool)
        n35 = local write "Error"(w70) -> ()
        n36 = local write "error"(w74) -> ()
        n37 = Bundle By Name(cluster=w72, "Error"=w70) -> (w71:T16)
        n38 = call <vilib>:"Add State(s) to Queue__JKI_lib_State_Machine.vi"("State(s) in Front (\"\")"="4461: RESET\nMacro: Exit", "State(s) in (\"\")"=w79) -> ("States Out"=w78:string)  [unwired: 13 in]
      }
      frame "Exit" {
        # "Do not put any code in this frame.\n(No errors that occur here will be handled.)"
        n39 = call <vilib>:"Add State(s) to Queue__JKI_lib_State_Machine.vi"("State(s) in (\"\")"=w84) -> ("States Out"=w83:string)  [unwired: 14 in]
      }
      frame "---------- Data ----------" {
        # "Do not put any code in this frame.\n(It is a separator no-op. You can make a copy of this frame to create a new Data frame)"
        n40 = call <vilib>:"Add State(s) to Queue__JKI_lib_State_Machine.vi"("State(s) in (\"\")"=w88) -> ("States Out"=w87:string)  [unwired: 14 in]
      }
      frame "Data: Initialize" {
        w89 = cluster{"Fs":dbl, "#s":dbl} {"Fs"=204800.0, "#s"=204800.0}  # sampling info
        w90 = waveform(dbl)[] []  # Ouput Signals
        w92 = waveform(dbl)[] []  # Input Signals
        w91 = waveform(dbl)[] []  # REF
        w93 = refnum<k21>[] []  # AO task
        w94 = refnum<k21>[] []  # AI task
        w95 = T18 {"Current VI Reference"=refnum, "Close Panel on Exit?"=FALSE}  # Core
        w97 = FALSE  # Error
        w96 = ""  # Your string data
        # "do not delete - used by framework"
        # "Expand Bundle to add new data elements to shift register data."
        # "Add new data here."
        # "Data names and types of shift register data are defined by this bundle."
        # "Initialize the shift-register data, here.\n(data names are defined by what you wire into the bundle function)"
        n41 = Bundle("Core"=w95, "Error"=w97, "Your string data"=w96, "AI task"=w94, "AO task"=w93, "Input Signals"=w92, "Ouput Signals"=w90, "REF"=w91, "sampling info"=w89) -> (w99:T16)  [unwired: 1 in]
        n42 = call <vilib>:"Add State(s) to Queue__JKI_lib_State_Machine.vi"("State(s) in (\"\")"=w101) -> ("States Out"=w100:string)  [unwired: 14 in]
      }
      frame "Data: Cleanup" {
        # "Cleanup any data and references, here.\n(this is called automatically, by the Macro: Exit)"
        n43 = Unbundle By Name(w102) -> ("Core.Current VI Reference"=w105:refnum<vi>)
        n44 = Close Reference(reference=w105, error in (no error)=w104) -> (error out=w103:errorcluster)
        n45 = call <vilib>:"Add State(s) to Queue__JKI_lib_State_Machine.vi"("State(s) in (\"\")"=w107) -> ("States Out"=w106:string)  [unwired: 14 in]
      }
      frame "---------- UI ----------" {
        # "Do not put any code in this frame.\n(It is a separator no-op. You can make a copy of this frame to create a new UI frame)"
        n46 = call <vilib>:"Add State(s) to Queue__JKI_lib_State_Machine.vi"("State(s) in (\"\")"=w111) -> ("States Out"=w110:string)  [unwired: 14 in]
      }
      frame "UI: Initialize" {
        w113 = FALSE ("EXIT")
        w117 = waveform(dbl)[][] [] ("History Data")
        # "empty Display charts"
        # "Initialize the User Interface, here.\n(this is called automatically, by the Macro: Init)"
        n47 = local write "error"(errorcluster {"status"=FALSE, "code"=0, "source"=""} ("error out")) -> ()
        n48 = local write "RESET"(w113) -> ()
        n49 = local write "EXIT"(w113) -> ()
        n50 = local write "Error"(w113) -> ()
        n51 = property on="Display X (or R)" class="WaveformChart (strict)"("History Data"=w117) -> ()  [unwired: 2 in, 2 out]
        n52 = property on="Display Y (or Theta)" class="WaveformChart (strict)"("History Data"=w117) -> ()  [unwired: 2 in, 2 out]
        n53 = local write "save time"(timestamp(0 s since 1904-01-01) ("save time")) -> ()
        n54 = call <vilib>:"Add State(s) to Queue__JKI_lib_State_Machine.vi"("State(s) in (\"\")"=w119) -> ("States Out"=w118:string)  [unwired: 14 in]
      }
      frame "UI: Cursor Set" {
        # "Argument"
        # "Set and Unset Cursor Busy.\n(Usage: \"UI: Cursor Set >> Busy|Idle\")"
        n55 = case shown="\"Busy\"" w121 {
          tunnel: w123 -> [w127 w129]
          tunnel: [w126 w128] -> w122
          frame "Idle", Default {
            n56 = call <vilib>:"Unset Busy.vi"("error in (no error)"=w127) -> ("error out"=w126:errorcluster)  [unwired: 10 in]
          }
          frame "Busy" {
            n57 = call <vilib>:"Set Busy.vi"("error in (no error)"=w129) -> ("error out"=w128:errorcluster)  [unwired: 9 in, 1 out]
          }
        }
        n58 = call <vilib>:"Add State(s) to Queue__JKI_lib_State_Machine.vi"("State(s) in (\"\")"=w125) -> ("States Out"=w124:string)  [unwired: 14 in]
      }
      frame "UI: Front Panel State" {
        # "Argument"
        # "Set Front Panel Open or Closed\n(Usage: \"UI: Front Panel State >> Open|Close\")"
        n59 = Unbundle By Name(w131) -> ("Core.Current VI Reference"=w133:refnum<vi>)
        n60 = case shown="\"Open\", Default" w132 {
          tunnel: w134 -> [w140 w153]
          tunnel: [w142 w154] -> w130
          tunnel: w133 -> [w141 w151]
          frame "Open", Default {
            n61 = property class="VI"(reference=w141, error in=w140) -> (reference out=w138:refnum<vi>, error out=w139:errorcluster, "Front Panel.Open"=w137:bool)
            n62 = case shown="True" w137 {
              tunnel: [w145 w148] -> w142
              tunnel: w139 -> [w144 w148]
              tunnel: w138 -> [w143 _]
              frame False {
                n63 = invoke class="VI" method="FP.Open"(reference=w143, error in=w144, "Activate"=TRUE, "State"=T14."Standard") -> (error out=w145:errorcluster)  [unwired: 1 in, 4 out]
              }
              frame True {
              }
            }
          }
          frame "Close" {
            n64 = property class="VI"(reference=w151, error in=w153) -> (reference out=w150:refnum<vi>, error out=w152:errorcluster, "Front Panel.Open"=w149:bool)
            n65 = case shown="True" w149 {
              tunnel: [w155 w158] -> w154
              tunnel: w152 -> [w155 w157]
              tunnel: w150 -> [_ w156]
              frame False {
              }
              frame True {
                n66 = invoke class="VI" method="FP.Close"(reference=w156, error in=w157) -> (error out=w158:errorcluster)  [unwired: 1 in, 2 out]
              }
            }
          }
        }
        n67 = call <vilib>:"Add State(s) to Queue__JKI_lib_State_Machine.vi"("State(s) in (\"\")"=w136) -> ("States Out"=w135:string)  [unwired: 14 in]
      }
      frame "---------- Macro ----------" {
        # "Do not put any code in this frame.\n(It is a separator no-op. You can make a copy of this frame to create a new Macro frame)"
        n68 = call <vilib>:"Add State(s) to Queue__JKI_lib_State_Machine.vi"("State(s) in (\"\")"=w162) -> ("States Out"=w161:string)  [unwired: 14 in]
      }
      frame "Macro: Initialize" {
        w164 = "Data: Initialize\nInitialize Core Data\nUI: Initialize\nUI: Front Panel State >> Open\n4461: SETUP"  # Data: Initialize Initialize Core Data UI: Initialize UI: Front Panel State >> Open 4461: SETUP
        # "Initialization Macro\n(This is called once, when the VI starts)"
        n69 = call <vilib>:"Add State(s) to Queue__JKI_lib_State_Machine.vi"("State(s) in Front (\"\")"=w164, "State(s) in (\"\")"=w167) -> ("States Out"=w166:string)  [unwired: 13 in]
      }
      frame "Macro: Exit" {
        w169 = FALSE ("EXIT")
        # "Exit Macro\n(This is called once, when the VI exits)"
        n70 = Unbundle By Name(w168) -> ("Core.Close Panel on Exit?"=w175:bool)
        n71 = local write "EXIT"(w169) -> ()
        n72 = local write "RESET"(w169) -> ()
        n73 = Select(t="UI: Front Panel State >> Close", s=w175, f="") -> (s? t:f=w172:string)
        n74 = call <vilib>:"Add State(s) to Queue__JKI_lib_State_Machine.vi"("State(s) in (\"\")"=w172, "State(s) at Back (\"\")"="Data: Cleanup\nExit") -> ("States Out"=w170:string)  [unwired: 13 in]
        n75 = call <vilib>:"Add State(s) to Queue__JKI_lib_State_Machine.vi"("State(s) in Front (\"\")"=w170, "State(s) in (\"\")"=w178) -> ("States Out"=w177:string)  [unwired: 13 in]
      }
      frame "---------- 4461----------" {
        n76 = call <vilib>:"Add State(s) to Queue__JKI_lib_State_Machine.vi"("State(s) in (\"\")"=w182) -> ("States Out"=w181:string)  [unwired: 14 in]
      }
      frame "4461: SETUP" {
        n77 = local read "Channels: AO"() -> (w206:T8)
        n78 = local read "Remote Mode"() -> (w191:bool)
        n79 = Unbundle By Name(w206) -> ("AO f (Hz)"=w184:dbl[])
        n80 = Unbundle By Name(w187) -> ("sampling info"=w188:cluster{"Fs":dbl, "#s":dbl})
        n81 = call <userlib>:"FGV - Remote.vi"("error in"=w193, "Function"=enum16{"write", "read"}."write", "Remote Mode"=w191) -> ("error out"=w192:errorcluster)  [unwired: 3 in, 1 out]
        n82 = Index Array(array=w184) -> (element=w183:dbl)  [unwired: 1 in]
        n83 = case shown="True" "auto block size" {
          tunnel: w188 -> [_ w213]
          tunnel: [w210 w214] -> w186
          tunnel: w183 -> [_ w212]
          frame False {
            n84 = local read "sampling info"() -> (w210:cluster{"Fs":i32, "#s":i32})
          }
          frame True {
            n85 = case shown="True" TRUE {
              tunnel: [w215 w228] -> w214
              tunnel: w213 -> [w215 w227]
              tunnel: w212 -> [_ w217]
              frame False {
                # "\"IV mode\""
              }
              frame True {
                n86 = Multiply(x="x", y=w217) -> (x*y=w226:dbl)
                n87 = In Range and Coerce(upper limit=204800.0, x=w226, lower limit=1000.0) -> (coerced(x)=w216:dbl)  [unwired: 1 out]
                n88 = call <userlib>:"Fs and Ns for integer periods.vi"("f_integer"=w217, "Fs"=w216) -> ("#s_integer"=w218:dbl, "Fs_integer"=w223:dbl)  [unwired: 8 in]
                n89 = In Range and Coerce(upper limit=204800.0, x=w223, lower limit=1000.0) -> (coerced(x)=w222:dbl)  [unwired: 1 out]
                n90 = Bundle By Name(cluster=w227, "Fs"=w222, "#s"=w218) -> (w228:cluster{"Fs":dbl, "#s":dbl})
                n91 = local write "sampling info"(w228) -> ()
              }
            }
          }
        }
        n92 = local read "Channels: Lockin"() -> (w196:T9)
        n93 = call <userlib>:"FGV - Configuration - lockin.vi"("error in"=w192, "Function"=enum16{"write", "read"}."write", "Channels: Lockin"=w196) -> ("error out"=w201:errorcluster)  [unwired: 3 in, 1 out]
        n94 = local read "Channels: AO"() -> (w195:T8)
        n95 = call <userlib>:"FGV - Configuration - Output.vi"("error in"=w201, "Function"=enum16{"write", "read"}."write", "Channels: AO"=w195) -> ("error out"=w200:errorcluster)  [unwired: 3 in, 1 out]
        n96 = call <userlib>:"FGV - Trigger.vi"("error in"=w200, "Function"=enum16{"write", "read"}."write", "Trigger"=TRUE) -> ("error out"=w189:errorcluster)  [unwired: 3 in, 1 out]
        n97 = local read "Gain"() -> (w194:dbl[])
        n98 = Bundle By Name(cluster=w187, "sampling info"=w186) -> (w185:T16)
        n99 = call <userlib>:"FGV - KH Gain.vi"("error in"=w189, "Function"=enum16{"write", "read"}."write", "Array"=w194) -> ("error out"=w197:errorcluster)  [unwired: 3 in, 1 out]
        n100 = call <vilib>:"Add State(s) to Queue__JKI_lib_State_Machine.vi"("State(s) in (\"\")"=w209, "State(s) at Back (\"\")"="4461: CREATE" ("State(s) at Back (\"\")")) -> ("States Out"=w208:string)  [unwired: 13 in]
      }
      frame "4461: CREATE" {
        w232 = 10178 items=["Finite Samples"=10178, "Continuous Samples"=10123] ("sample mode")
        w231 = 10123 items=["Finite Samples"=10178, "Continuous Samples"=10123] ("sample mode")
        # "(finite?)"
        n101 = local read "AO Configuration"() -> (w237:T6)
        n102 = local read "AI Configuration"() -> (w239:T7)
        n103 = local read "AI Buffer Size (S)"() -> (w245:i32)
        n104 = Unbundle By Name(w234) -> ("sampling info"=w235:cluster{"Fs":dbl, "#s":dbl})
        n105 = local read "Channels: AO"() -> (w246:T8)
        n106 = local read "simulate?"() -> (w233:bool)
        n107 = local read "IV curves?"() -> (w230:bool)
        n108 = Select(t=w232, s=w230, f=w231) -> (s? t:f=w229:i32)
        n109 = case shown="False" w233 {
          tunnel: w239 -> [w259 _]
          tunnel: w237 -> [w258 _]
          tunnel: [w257 w278] -> w244
          tunnel: w235 -> [w256 _]
          tunnel: [w255 w278] -> w243
          tunnel: w245 -> [w254 _]
          tunnel: [w253 dbl[] [] ("phase log")] -> w238
          tunnel: w246 -> [w252 _]
          tunnel: w240 -> [w251 w273]
          tunnel: [w250 w272] -> w236
          tunnel: w229 -> [w249 _]
          frame False {
            n110 = disable-structure shown="Default" {
              disable-tunnel: w259 -> [w270 _]
              disable-tunnel: w258 -> [w269 _]
              disable-tunnel: [w268 _] -> w257
              disable-tunnel: w256 -> [w265 _]
              disable-tunnel: [w267 _] -> w255
              disable-tunnel: w254 -> [w263 _]
              disable-tunnel: [w264 _] -> w253
              disable-tunnel: w252 -> [w266 _]
              disable-tunnel: w251 -> [w262 _]
              disable-tunnel: [w261 _] -> w250
              disable-tunnel: w249 -> [w260 _]
              frame condition #0 (active) {
                n111 = call <userlib>:"4461 - Create IO Channels Parallel.vi"("sample mode"=w260, "error in"=w262, "AI Buffer Size (S)"=w263, "sampling info"=w265, "AO"=w266, "AO Configuration"=w269, "AI Configuration"=w270) -> ("AO Task"=w267:refnum<k21>[], "AI task"=w268:refnum<k21>[], "error out"=w261:errorcluster, "phase log"=w264:dbl[])  [unwired: 1 in]
              }
              frame condition #1 {
              }
            }
          }
          frame True {
            w278 = refnum<k21>[] [] ("AI task")
            # "simulate mode"
            n112 = Initialize Array(1.0 ("element"), 8 ("dimension size")) -> (w271:dbl[])
            n113 = call <userlib>:"FGV - KH Gain.vi"("error in"=w273, "Function"=enum16{"write", "read"}."write", "Array"=w271) -> ("error out"=w272:errorcluster)  [unwired: 3 in, 1 out]
            n114 = local write "Gain"(w271) -> ()
          }
        }
        n115 = local write "phase log"(w238) -> ()
        n116 = Bundle By Name(cluster=w234, "AI task"=w244, "AO task"=w243) -> (w242:T16)
        n117 = call <vilib>:"Add State(s) to Queue__JKI_lib_State_Machine.vi"("State(s) in (\"\")"=w248, "State(s) at Back (\"\")"="4461: FGV" ("State(s) at Back (\"\")")) -> ("States Out"=w247:string)  [unwired: 13 in]
      }
      frame "4461: FGV" {
        n118 = call <userlib>:"FGV - Remote.vi"("error in"=w290, "Function"=enum16{"write", "read"}."read") -> ("error out"=w289:errorcluster, "Remote Mode"=w285:bool)  [unwired: 4 in]
        n119 = local write "Remote Mode"(w285) -> ()
        n120 = call <userlib>:"FGV - Configuration - Output.vi"("error in"=w289, "Function"=enum16{"write", "read"}."read") -> ("error out"=w292:errorcluster, "Channels: AO 2"=w281:T8)  [unwired: 4 in]
        n121 = local read "Channels: Lockin"() -> (w282:T9)
        n122 = local read "Channels: AO"() -> (w283:T8)
        n123 = call <userlib>:"FGV - Configuration - lockin.vi"("error in"=w292, "Function"=enum16{"write", "read"}."read") -> ("error out"=w288:errorcluster, "Channels: Lockin 2"=w284:T9)  [unwired: 4 in]
        n124 = Select(t=w281, s=w285, f=w283) -> (s? t:f=w280:T8)
        n125 = Select(t=w284, s=w285, f=w282) -> (s? t:f=w279:T9)
        n126 = local write "Channels: AO"(w280) -> ()
        n127 = local write "Channels: Lockin"(w279) -> ()
        n128 = call <userlib>:"FGV - Configuration - lockin.vi"("Function"=enum16{"write", "read"}."write", "Channels: Lockin"=w279) -> ()  [unwired: 4 in, 2 out]
        n129 = call <userlib>:"FGV - Configuration - Output.vi"("Function"=enum16{"write", "read"}."write", "Channels: AO"=w280) -> ()  [unwired: 4 in, 2 out]
        n130 = call <userlib>:"FGV - KH Gain.vi"("error in"=w288, "Function"=enum16{"write", "read"}."read") -> ("error out"=w294:errorcluster, "Array 2"=w293:dbl[])  [unwired: 4 in]
        n131 = local write "Gain"(w293) -> ()
        n132 = call <vilib>:"Add State(s) to Queue__JKI_lib_State_Machine.vi"("State(s) in (\"\")"=w299, "State(s) at Back (\"\")"="4461: DATA" ("State(s) at Back (\"\")")) -> ("States Out"=w300:string)  [unwired: 13 in]
      }
      frame "4461: DATA" {
        (unwired) waveform(dbl)[] [] ("Array out")
        n133 = Unbundle By Name(w325) -> ("sampling info"=w322:cluster{"Fs":dbl, "#s":dbl}, "AI task"=w324:refnum<k21>[])
        n134 = First Call?() -> (First Call?: T/F=w310:bool)
        n135 = local read "measure offset"() -> (w319:bool)
        n136 = local read "Channels: AO"() -> (w307:T8)
        n137 = Unbundle By Name(w307) -> ("AO amp (V)"=w304:dbl[])
        n138 = Array Size(array=w304) -> (size(s)=w305:i32)
        n139 = Initialize Array(0.0 ("element"), w305) -> (w302:dbl[])
        n140 = local read "Channels: Lockin"() -> (w317:T9)
        n141 = local read "reset signal"() -> (w320:bool)
        n142 = Bundle By Name(cluster=w307, "AO amp (V)"=w302) -> (w306:T8)
        n143 = Or(x=w310, y=w320) -> (x .or. y?=w309:bool)
        n144 = Select(t=w306, s=w319, f=w307) -> (s? t:f=w318:T8)
        n145 = call <userlib>:"4461 - Create AO waveforms.vi"("error in (no error)"=w337, "sampling info"=w322, "reset signal"=w309, "AO"=w318) -> ("error out"=w316:errorcluster, "phase out"=w312:dbl[], "AO Array"=w315:waveform(dbl)[])  [unwired: 4 in, 1 out]
        n146 = call <userlib>:"4461 - Create Reference Waveforms.vi"("error in (no error)"=w337, "sampling info"=w322, "reset signal"=w309, "Lockin"=w317) -> ("error out"=w328:errorcluster, "AO Array"=w326:waveform(dbl)[])  [unwired: 4 in, 2 out]
        n147 = local read "simulate?"() -> (w314:bool)
        n148 = call-poly <userlib>:"Empty Array__ogtk.vi"("Array"=w324) -> ("Empty Array?"=w323:bool)  [unwired: 8 in]
        n149 = local write "phase log"(w312) -> ()
        n150 = Or(x=w323, y=w314) -> (x .or. y?=w313:bool)
        n151 = case shown="False" w313 {
          tunnel: [w350 w363] -> w321
          tunnel: w315 -> [w344 w361]
          tunnel: w322 -> [w345 w360]
          tunnel: w325 -> [w347 _]
          tunnel: w316 -> [w346 w362]
          tunnel: [w348 w362] -> w336
          tunnel: [w343 w361] -> w311
          tunnel: FALSE -> [w341 _]
          frame False {
            n152 = Unbundle By Name(w347) -> ("AI task"=w349:refnum<k21>[], "AO task"=w342:refnum<k21>[])
            n153 = disable-structure shown="Default" {
              disable-tunnel: [w352 _] -> w350
              disable-tunnel: w344 -> [w353 w359]
              disable-tunnel: w345 -> [w354 _]
              disable-tunnel: w349 -> [w356 _]
              disable-tunnel: w346 -> [w358 _]
              disable-tunnel: [w357 _] -> w348
              disable-tunnel: [w353 w359] -> w343
              disable-tunnel: w342 -> [w355 _]
              disable-tunnel: w341 -> [w351 _]
              frame condition #0 (active) {
                n154 = call <userlib>:"4461 - AI AND AI - Read AND Write.vi"("Reset"=w351, "AO Array"=w353, "error in (no error)"=w358, "sampling info"=w354, "AO Task"=w355, "AI task"=w356) -> ("error out"=w357:errorcluster, "Input Signals"=w352:waveform(dbl)[])  [unwired: 4 in]
              }
              frame condition #1 {
              }
            }
          }
          frame True {
            n155 = call <userlib>:"4461 Sim - Noise.vi"("data"=w361, "sampling info"=w360) -> ("Data"=w363:waveform(dbl)[])  [unwired: 5 in]
          }
        }
        n156 = Index Array(array=w321) -> (element=w334:waveform(dbl))  [unwired: 1 in]
        n157 = Bundle By Name(cluster=w325, "Input Signals"=w321, "Ouput Signals"=w311, "REF"=w326) -> (w338:T16)
        n158 = Unbundle By Name(w334) -> ("Y"=w333:dbl[])
        n159 = local write "time since trigger"(0.0 ("time since trigger")) -> ()
        n160 = call-poly <userlib>:"Empty Array__ogtk.vi"("Array"=w333) -> ("Empty Array?"=w331:bool)  [unwired: 8 in]
        n161 = Merge Errors(w336, w328) -> (w335:errorcluster)
        n162 = Select(t="4461: RESET" ("State(s) at Back (\"\")"), s=w331, f="4461: MOD" ("State(s) at Back (\"\")")) -> (s? t:f=w330:string)
        n163 = call <vilib>:"Add State(s) to Queue__JKI_lib_State_Machine.vi"("State(s) in (\"\")"=w340, "State(s) at Back (\"\")"=w330) -> ("States Out"=w339:string)  [unwired: 13 in]
      }
      frame "4461: MOD" {
        w364 = TRUE ("averaging")
        n164 = Unbundle By Name(w366) -> ("Ouput Signals"=w378:waveform(dbl)[], "Input Signals"=w388:waveform(dbl)[], "REF"=w377:waveform(dbl)[])
        n165 = local read "decimating factor"() -> (w369:i32)
        n166 = call <userlib>:"decimate_waveforms.vi"("decimating factor"=w369, "averaging"=w364, "error in (no error)"=w383, "Input Signal"=w378) -> ("error out"=w382:errorcluster, "Decimated Waveforms"=w368:waveform(dbl)[])  [unwired: 6 in]
        n167 = call <userlib>:"decimate_waveforms.vi"("decimating factor"=w369, "averaging"=w364, "error in (no error)"=w383, "Input Signal"=w388) -> ("error out"=w385:errorcluster, "Decimated Waveforms"=w375:waveform(dbl)[])  [unwired: 6 in]
        n168 = call <userlib>:"decimate_waveforms.vi"("decimating factor"=w369, "averaging"=w364, "error in (no error)"=w383, "Input Signal"=w377) -> ("error out"=w384:errorcluster, "Decimated Waveforms"=w367:waveform(dbl)[])  [unwired: 6 in]
        n169 = local read "offsets"() -> (w389:dbl[])
        n170 = Subtract(x=w375, y=w389) -> (x-y=w374:waveform(dbl)[])
        n171 = Merge Errors(w382, w385, w384) -> (w380:errorcluster)
        n172 = case shown="False" "60 Hz prefilter" {
          tunnel: w374 -> [w397 w399]
          tunnel: [w397 w398] -> w373
          frame False {
          }
          frame True {
            n173 = call <userlib>:"Prefilter_60Hz_Notch.vi"("Array"=w399) -> ("Array 2"=w398:waveform(dbl)[])  [unwired: 10 in]
          }
        }
        n174 = local read "measure offset"() -> (w381:bool)
        n175 = local read "zero offset"() -> (w379:bool)
        n176 = Index Array(array=w367) -> (element=w387:waveform(dbl))  [unwired: 1 in]
        n177 = case shown="False" "LP prefilter" {
          tunnel: w373 -> [w393 w396]
          tunnel: [w393 w395] -> w372
          tunnel: "LP cutoff (Hz)" -> [_ w394]
          frame False {
          }
          frame True {
            n178 = call <userlib>:"Prefilter_LP.vi"("high cutoff freq [Hz]"=w394, "Array"=w396) -> ("Array 2"=w395:waveform(dbl)[])  [unwired: 9 in]
          }
        }
        n179 = Unbundle By Name(w387) -> ("dt"=w386:dbl)
        n180 = local write "dt"(w386) -> ()
        n181 = case shown="False" w381 {
          tunnel: w366 -> [w403 w408]
          frame False {
            n182 = Unbundle By Name(w403) -> ("Input Signals"=w402:waveform(dbl)[])
            n183 = for {
              tunnel: w402 -> [w405] mode=indexing
              tunnel: [w404] -> w401 mode=indexing
              n184 = call-poly <vilib>:"Mean.vi"("X"=w405) -> ("mean"=w404:dbl)  [unwired: 1 out]
            }
            n185 = local write "mean"(w401) -> ()
          }
          frame True {
            n186 = Unbundle By Name(w408) -> ("Input Signals"=w407:waveform(dbl)[])
            n187 = for {
              tunnel: w407 -> [w410] mode=indexing
              tunnel: [w409] -> w406 mode=indexing
              n188 = call-poly <vilib>:"Mean.vi"("X"=w410) -> ("mean"=w409:dbl)  [unwired: 1 out]
            }
            n189 = local write "offsets"(w406) -> ()
            n190 = local write "mean"(w406) -> ()
          }
        }
        n191 = case shown="True" w379 {
          frame False {
          }
          frame True {
            n192 = local write "offsets"(dbl[] [0.0, 0.0, 0.0, 0.0, 0.0, 0.0, 0.0, 0.0] ("offsets")) -> ()
          }
        }
        n193 = Bundle By Name(cluster=w366, "Ouput Signals"=w368, "Input Signals"=w372, "REF"=w367) -> (w390:T16)
        n194 = call <vilib>:"Add State(s) to Queue__JKI_lib_State_Machine.vi"("State(s) in (\"\")"=w392, "State(s) at Back (\"\")"="4461: PHASE" ("State(s) at Back (\"\")")) -> ("States Out"=w391:string)  [unwired: 13 in]
      }
      frame "4461: PHASE" {
        n195 = local read "Results\n(X, Y, R, Theta, mean)"() -> (w423:dbl[][])
        n196 = local read "autophase?\n(experimental)"() -> (w422:bool)
        n197 = local read "phase log"() -> (w424:dbl[])
        n198 = local read "Channels: Lockin"() -> (w420:T9)
        n199 = local read "Channels: AO"() -> (w419:T8)
        n200 = call <userlib>:"lockin - Set all f same.vi"("all  frequencies same?"="all  f same?", "Lockin"=w420, "AO"=w419) -> ("Lockin 2"=w417:T9, "AO 2"=w416:T8)  [unwired: 7 in]
        n201 = call <userlib>:"lockin - Set REF phase equals zero.vi"("reset REF phi to zero"="reset REF phi to zero", "Lockin"=w417, "AO"=w416) -> ("Lockin 2"=w412:T9, "AO 2"=w418:T8)  [unwired: 7 in]
        n202 = case shown="False" w422 {
          tunnel: w424 -> [_ w433]
          tunnel: w423 -> [_ w432]
          tunnel: w412 -> [w428 w430]
          tunnel: [w428 w429] -> w413
          frame False {
          }
          frame True {
            # "do this for EACH lockin...\n- replace PID array with PID SV\n-  advance \"results\" by 8?\n- this should go BEFORE REF\nwaveform is generated"
            n203 = Index Array(array=w432, index (col)=3 ("index (row)")) -> (element=w435:dbl[])  [unwired: 1 in]
            n204 = call <userlib>:"Simple PID Array.vi"("D"="D", "I"="I", "P"="P", "process variable"=w435) -> ("output value"=w439:dbl[])  [unwired: 7 in]
            n205 = Subtract(x=w433, y=w439) -> (x-y=w431:dbl[])
            n206 = Bundle By Name(cluster=w430, "REF phi (deg)"=w431) -> (w429:T9)
          }
        }
        n207 = local write "Channels: AO"(w418) -> ()
        n208 = local write "Channels: Lockin"(w413) -> ()
        n209 = call <vilib>:"Add State(s) to Queue__JKI_lib_State_Machine.vi"("State(s) in (\"\")"=w427, "State(s) at Back (\"\")"="4461: LOCKIN" ("State(s) at Back (\"\")")) -> ("States Out"=w426:string)  [unwired: 13 in]
      }
      frame "4461: LOCKIN" {
        n210 = event shown="[0] Timeout" {
          selector: _ -> [_ _ _ _ _ _]
          dyn-events: _ -> [_ _ _ _ _ _]
          timeout: 0 -> [_ _ _ _ _ _]
          tunnel: w445 -> [w512 w513 w522 w526 w532 w540]
          tunnel: [w511 w514 w524 w528 w534 w539] -> w442
          tunnel: w446 -> [w509 w516 w523 w529 w535 w537]
          tunnel: [w510 w517 w525 w527 w531 w538] -> w443
          tunnel: w444 -> [w510 w518 w525 w527 w531 w538]
          tunnel: [w509 w516 w523 w529 w535 w537] -> w441
          event Timeout {
            n211 = event-data() -> ()  [unwired: 1 in, 1 out]
            n212 = Unbundle By Name(w509) -> ("Ouput Signals"=w450:waveform(dbl)[], "Input Signals"=w465:waveform(dbl)[], "REF"=w451:waveform(dbl)[], "sampling info"=w483:cluster{"Fs":dbl, "#s":dbl})
            n213 = local read "TC (s)"() -> (w508:dbl)
            n214 = local read "mean"() -> (w499:dbl[])
            n215 = local read "order"() -> (w507:i32)
            n216 = local read "Gain"() -> (w493:dbl[])
            n217 = Select(t=w450, s="Output signals?", f=w451) -> (s? t:f=w449:waveform(dbl)[])
            n218 = Divide(x=w465, y=w493) -> (x/y=w466:waveform(dbl)[])
            n219 = call <userlib>:"Display n or dt.vi"("Display n?"="Display n?", "Input Waveforms"=w449) -> ("Output Waveforms"=w474:waveform(dbl)[])  [unwired: 9 in]
            n220 = call <userlib>:"Display n or dt.vi"("Display n?"="Display n?", "Input Waveforms"=w465) -> ("Output Waveforms"=w476:waveform(dbl)[])  [unwired: 9 in]
            n221 = Divide(x=w499, y=w493) -> (x/y=w498:dbl[])
            n222 = call <userlib>:"decimate_waveforms.vi"("decimating factor"="decimate graph", "averaging"=FALSE, "Input Signal"=w474) -> ("Decimated Waveforms"=→"Reference Graph":waveform(dbl)[])  [unwired: 7 in, 1 out]
            n223 = Index Array(array=w466) -> (element=w462:waveform(dbl))  [unwired: 1 in]
            n224 = call <userlib>:"decimate_waveforms.vi"("decimating factor"="decimate graph", "averaging"=FALSE, "Input Signal"=w476) -> ("Decimated Waveforms"=→"Signals Graph":waveform(dbl)[])  [unwired: 7 in, 1 out]
            n225 = Get Date/Time In Seconds() -> (seconds since 1Jan1904=w456:timestamp)
            n226 = Unbundle By Name(w462) -> ("t0"=w486:timestamp)
            n227 = local write "current time"(w456) -> ()
            n228 = local read "save time"() -> (w472:timestamp)
            n229 = call <userlib>:"4461 - Lockin Engine.vi"("order"=w507, "TC (s)"=w508, "sampling info"=w483, "Reference In"=w451, "Signal in"=w466) -> ("filter fC (Hz)"=w447:dbl, "Results (X,Y,R,Theta)"=w501:dbl[][])  [unwired: 5 in]
            n230 = Transpose 2D Array(2D array=w501) -> (transposed array=w491:dbl[][])
            n231 = Build Array (concatenate)(w491, w498) -> (w500:dbl[][])
            n232 = Format Date/Time String(time format string (%c)="%S", seconds (now)=w456) -> (date/time string=w454:string)  [unwired: 1 in]
            n233 = call <userlib>:"FGV - Signals - Input.vi"("Function"=enum16{"write", "read"}."write", "input signal"=w466) -> ()  [unwired: 4 in, 2 out]
            n234 = local read "Channel"() -> (w448:dbl)
            n235 = local write "filter fC (Hz)"(w447) -> ()
            n236 = Subtract(x=w456, y=w472) -> (x-y=w457:dbl)
            n237 = local read "Display"() -> (w506:enum16{"X and Y", "R and Theta"})
            n238 = Transpose 2D Array(2D array=w500) -> (transposed array=w467:dbl[][])
            "Results\n(X, Y, R, Theta, mean)" <- w467
            n239 = call <userlib>:"FGV - Signals - Output.vi"("Function"=enum16{"write", "read"}."write", "input signal"=w450) -> ()  [unwired: 4 in, 2 out]
            n240 = Fract/Exp String To Number(string=w454) -> (number=→"Gauge":dbl)  [unwired: 3 in, 1 out]
            n241 = local read "Tab Control 2"() -> (w495:T1)
            n242 = call <userlib>:"format display.vi"("Channel"=w448, "Display"=w506, "Results (X,Y,R,Theta)"=w501, "t0"=w486) -> ("X/R"=→"X or R":dbl, "Array 2"=→"XY Graph":cluster{dbl[], dbl[]}[], "Y/Theta Array"=→"Display Y (or Theta)":waveform(dbl)[], "X/R Array"=→"Display X (or R)":waveform(dbl)[], "Y/R"=→"Y or Theta":dbl)  [unwired: 3 in]
            n243 = Greater?(x=w457, y="save interval (s)") -> ()  [unwired: 1 out]
            n244 = call <userlib>:"FGV - Lockin Results.vi"("Function"=enum16{"write", "read"}."write", "Input Signals"=w467) -> ()  [unwired: 4 in, 2 out]
            n245 = local read "Wait on Trigger"() -> (w502:bool)
            n246 = Equal?(x=w495, y=T15."PS" ("Tab Control 2")) -> (x = y?=w497:bool)
            n247 = Equal?(x=w495, y=T15."FFT" ("Tab Control 2")) -> (x = y?=w478:bool)
            n248 = local read "IV curves?"() -> (w459:bool)
            n249 = Or(x=w478, y=w497) -> (x .or. y?=w496:bool)
            n250 = Select(t="4461: TRIGGER" ("State(s) at Back (\"\")"), s=w502, f="4461: FGV" ("State(s) at Back (\"\")")) -> (s? t:f=w489:string)
            n251 = Select(t="4461: FFT" ("State(s) at Back (\"\")"), s=w496, f=w489) -> (s? t:f=w469:string)
            n252 = Select(t="4461: SAVE", s=FALSE, f=w469) -> (s? t:f=w461:string)
            n253 = Select(t="4461: EXIT\nMacro: Exit", s=w459, f=w461) -> (s? t:f=w460:string)
            n254 = call <vilib>:"Add State(s) to Queue__JKI_lib_State_Machine.vi"("State(s) in (\"\")"=w512, "State(s) at Back (\"\")"=w460) -> ("States Out"=w511:string)  [unwired: 13 in]
          }
          event "Remote Mode": Value Change {
            n255 = event-data() -> ()  [unwired: 1 in, 6 out]
            n256 = local read "Remote Mode"() -> (w520:bool)
            n257 = call <userlib>:"FGV - Remote.vi"("error in"=w518, "Function"=enum16{"write", "read"}."write", "Remote Mode"=w520) -> ("error out"=w517:errorcluster)  [unwired: 3 in, 1 out]
            n258 = call <vilib>:"Add State(s) to Queue__JKI_lib_State_Machine.vi"("State(s) in (\"\")"=w513, "State(s) at Back (\"\")"="4461: FGV" ("State(s) at Back (\"\")")) -> ("States Out"=w514:string)  [unwired: 13 in]
          }
          event "simulate?": Value Change {
            n259 = event-data() -> ()  [unwired: 1 in, 6 out]
            n260 = call <vilib>:"Add State(s) to Queue__JKI_lib_State_Machine.vi"("State(s) in (\"\")"=w522, "State(s) at Back (\"\")"="4461: RESET") -> ("States Out"=w524:string)  [unwired: 13 in]
          }
          event "Save Data": Value Change {
            n261 = event-data() -> ()  [unwired: 1 in, 6 out]
            n262 = call <vilib>:"Add State(s) to Queue__JKI_lib_State_Machine.vi"("State(s) in (\"\")"=w526, "State(s) at Back (\"\")"="4461: SAVE") -> ("States Out"=w528:string)  [unwired: 13 in]
          }
          event "RESET": Value Change {
            n263 = event-data() -> ()  [unwired: 1 in, 6 out]
            n264 = call <vilib>:"Add State(s) to Queue__JKI_lib_State_Machine.vi"("State(s) in (\"\")"=w532, "State(s) at Back (\"\")"="4461: RESET") -> ("States Out"=w534:string)  [unwired: 13 in]
          }
          event "EXIT": Value Change {
            (unwired) "4461: SETUP"
            (unwired) "4461: RESET"
            # "Add other events to reset lockin (4461: RESET --> 4461 SETUP)"
            # "Exit Button Value Change (pressed) Event\n(this executes Macro: Exit to terminate the VI)"
            n265 = event-data() -> ()  [unwired: 1 in, 1 out]
            n266 = call <vilib>:"Add State(s) to Queue__JKI_lib_State_Machine.vi"("State(s) in (\"\")"=w540, "State(s) at Back (\"\")"="4461: EXIT\nMacro: Exit") -> ("States Out"=w539:string)  [unwired: 13 in]
          }
        }
      }
      frame "4461: FFT" {
        n267 = Unbundle By Name(w562) -> ("Input Signals"=w541:waveform(dbl)[])
        n268 = local read "Gain"() -> (w560:dbl[])
        n269 = Divide(x=w541, y=w560) -> (x/y=w549:waveform(dbl)[])
        n270 = property on="PS dB" class="WFGraph (strict)"("Active Cursor"=u32 1) -> ("Cursor.Cursor X"=w554:dbl)  [unwired: 2 in, 2 out]
        n271 = property on="PS dB" class="WFGraph (strict)"("Active Cursor"=u32 0) -> ("Cursor.Cursor X"=w555:dbl)  [unwired: 2 in, 2 out]
        n272 = call-poly <vilib>:"FFT Power Spectrum and PSD.vi"("window parameter"="window parameter", "export mode"="export mode", "averaging parameters"="averaging parameters", "restart averaging (F)"="restart averaging (F)", "dB On (F)"=TRUE, "window"="window", "time signals"=w549) -> ("averages completed"=→"averages\ncompleted":dbl, "averaging done"=→"averaging done":bool, "Power Spectrum / PSD"=w557:cluster{"f0":dbl, "df":dbl, "magnitude":dbl[]}[])  [unwired: 1 in, 1 out]
        "PS dB" <- w557
        n273 = for {
          tunnel: w557 -> [w582] mode=indexing
          tunnel: [w577] -> w556 mode=indexing
          n274 = Unbundle By Name(w582) -> ("df"=w584:dbl, "magnitude"=w583:dbl[])  [unwired: 1 out]
          n275 = Bundle By Name("dt"=w584, "Y"=w583) -> (w581:waveform(dbl))  [unwired: 1 in]
          n276 = call-poly <vilib>:"Waveform to XY Pairs.vi"("waveform in"=w581) -> ("XY pairs"=w580:cluster{"x":timestamp, "y":dbl}[])  [unwired: 8 in, 2 out]
          n277 = for {
            tunnel: w580 -> [w588] mode=indexing
            tunnel: [w586] -> w578 mode=indexing
            tunnel: [w585] -> w579 mode=indexing
            n278 = Unbundle(w588) -> ("x"=w587:timestamp, "y"=w586:dbl)
            n279 = To Double Precision Float(number=w587) -> (double precision float=w585:dbl)
          }
          n280 = Bundle(w579, w578) -> (w577:cluster{dbl[], dbl[]})  [unwired: 1 in]
        }
        n281 = Build Array(w555, w554) -> (w553:dbl[])
        n282 = for {
          tunnel: w556 -> [w576] mode=indexing
          tunnel: w553 -> [w575]
          tunnel: [w567] -> w552 mode=indexing
          n283 = Array Max & Min(array=w575) -> (max value=w574:dbl, min value=w572:dbl)  [unwired: 2 out]
          n284 = Unbundle(w576) -> (w573:dbl[], w571:dbl[])
          n285 = Threshold 1D Array(2:w574, 3:w573) -> (0:w570:dbl)  [unwired: 1 in]
          n286 = Threshold 1D Array(2:w572, 3:w573) -> (0:w569:dbl)  [unwired: 1 in]
          n287 = Subtract(x=w570, y=w569) -> (x-y=w568:dbl)
          n288 = Array Subset(array=w571, index=w569, length=w568) -> (w566:dbl[])
          n289 = Add Array Elements(numeric array=w566) -> (sum=w567:dbl)
        }
        n290 = Build Array(w552) -> (→"PS Chart":dbl[][])
        n291 = call <vilib>:"Add State(s) to Queue__JKI_lib_State_Machine.vi"("State(s) in (\"\")"=w565, "State(s) at Back (\"\")"="4461: FGV" ("State(s) at Back (\"\")")) -> ("States Out"=w563:string)  [unwired: 13 in]
      }
      frame "4461: TRIGGER" {
        # "Wait for Trigger signal from other VI"
        n292 = Get Date/Time In Seconds() -> (seconds since 1Jan1904=w595:timestamp)
        n293 = while {
          tunnel: w595 -> [w611]
          tunnel: [FALSE ("Trigger")] -> w594
          tunnel: w592 -> [w603]
          tunnel: [w602] -> w591
          stop <- w608 stop-if-true
          # "Initiate trigger (acquire data) if wating longer\nthan 10 seconds"
          n294 = Get Date/Time In Seconds() -> (seconds since 1Jan1904=w612:timestamp)
          n295 = Wait (ms)(milliseconds to wait=u32 100) -> ()  [unwired: 1 out]
          n296 = Subtract(x=w612, y=w611) -> (x-y=w599:dbl)
          n297 = Greater?(x=w599, y=10.0) -> (0:w609:bool)
          n298 = call <userlib>:"FGV - Trigger.vi"("error in"=w603, "Function"=enum16{"write", "read"}."read") -> ("error out"=w602:errorcluster, "Trigger 2"=w605:bool)  [unwired: 4 in]
          n299 = local write "time since trigger"(w599) -> ()
          n300 = local read "Wait on Trigger"() -> (w600:bool)
          n301 = Not(x=w600) -> (.not. x?=w601:bool)
          n302 = Compound Arithmetic op=OR(w601, w609, w605) -> (w608:bool)
        }
        n303 = call <userlib>:"FGV - Trigger.vi"("error in"=w591, "Function"=enum16{"write", "read"}."write", "Trigger"=w594) -> ("error out"=w590:errorcluster)  [unwired: 3 in, 1 out]
        n304 = call <vilib>:"Add State(s) to Queue__JKI_lib_State_Machine.vi"("State(s) in (\"\")"=w598, "State(s) at Back (\"\")"="4461: FGV" ("State(s) at Back (\"\")")) -> ("States Out"=w597:string)  [unwired: 13 in]
      }
      frame "4461: SAVE" {
        w614 = "FFT" ("filename")
        w613 = "signal" ("filename")
        # "Wait for Trigger signal from other VI"
        n305 = local read "PS dB"() -> (w632:cluster{"f0":dbl, "df":dbl, "magnitude":dbl[]}[])
        n306 = Get Date/Time In Seconds() -> (seconds since 1Jan1904=w622:timestamp)
        n307 = for {
          tunnel: w632 -> [w652] mode=indexing
          tunnel: [w647] -> w627 mode=indexing
          n308 = Unbundle By Name(w652) -> ("df"=w654:dbl, "magnitude"=w653:dbl[])  [unwired: 1 out]
          n309 = Bundle By Name("dt"=w654, "Y"=w653) -> (w651:waveform(dbl))  [unwired: 1 in]
          n310 = call-poly <vilib>:"Waveform to XY Pairs.vi"("waveform in"=w651) -> ("XY pairs"=w650:cluster{"x":timestamp, "y":dbl}[])  [unwired: 8 in, 2 out]
          n311 = for {
            tunnel: w650 -> [w658] mode=indexing
            tunnel: [w656] -> w648 mode=indexing
            tunnel: [w655] -> w649 mode=indexing
            n312 = Unbundle(w658) -> ("x"=w657:timestamp, "y"=w656:dbl)
            n313 = To Double Precision Float(number=w657) -> (double precision float=w655:dbl)
          }
          n314 = Bundle(w649, w648) -> (w647:cluster{dbl[], dbl[]})  [unwired: 1 in]
        }
        n315 = local read "path"() -> (w619:path)
        n316 = local write "save time"(w622) -> ()
        n317 = call <userlib>:"FGV - Signals - Input.vi"("error in"=w624, "Function"=enum16{"write", "read"}."read") -> ("error out"=w625:errorcluster, "input signal"=w631:waveform(dbl)[])  [unwired: 4 in]
        n318 = for {
          tunnel: [w639] -> w630 mode=indexing
          tunnel: w631 -> [w638] mode=indexing
          n319 = call-poly <vilib>:"Waveform to XY Pairs.vi"("waveform in"=w638) -> ("XY pairs"=w642:cluster{"x":timestamp, "y":dbl}[])  [unwired: 8 in, 2 out]
          n320 = for {
            tunnel: w642 -> [w646] mode=indexing
            tunnel: [w644] -> w640 mode=indexing
            tunnel: [w643] -> w641 mode=indexing
            n321 = Unbundle(w646) -> ("x"=w645:timestamp, "y"=w644:dbl)
            n322 = To Double Precision Float(number=w645) -> (double precision float=w643:dbl)
          }
          n323 = Bundle(w641, w640) -> (w639:cluster{dbl[], dbl[]})  [unwired: 1 in]
        }
        n324 = Format Date/Time String(time format string (%c)="%Y-%m-%d", seconds (now)=w622) -> (date/time string=w620:string)  [unwired: 1 in]
        n325 = Build Path(base path=w619, name or relative path=w620) -> (appended path=w617:path)
        n326 = Build Path(base path=w617, name or relative path=w613) -> (appended path=w616:path)
        n327 = call <userlib>:"LV to ITX XY AutoPlot.vi"("filename"=w613, "path"=w616, "Notes"="Notes", "XY Array"=w630, "wavenames (.Vx, etc)"=string[] ["ch0", "ch1", "ch2", "ch3", "ch4", "ch5", "ch6", "ch7"]) -> ()  [unwired: 10 in, 1 out]
        n328 = Build Path(base path=w617, name or relative path=w614) -> (appended path=w615:path)
        n329 = local write "Save Data"(FALSE ("SAVE DATA")) -> ()
        n330 = call <userlib>:"LV to ITX XY AutoPlot.vi"("filename"=w614, "path"=w615, "Notes"="Notes", "XY Array"=w627, "wavenames (.Vx, etc)"=string[] ["FFT0", "FFT1", "FFT2", "FFT3", "FFT4", "FFT5", "FFT6", "FFT7"], "X,Y Log"=i32[] [1, 1]) -> ()  [unwired: 9 in, 1 out]
        n331 = call <vilib>:"Add State(s) to Queue__JKI_lib_State_Machine.vi"("State(s) in (\"\")"=w637, "State(s) at Back (\"\")"="4461: FGV" ("State(s) at Back (\"\")")) -> ("States Out"=w636:string)  [unwired: 13 in]
      }
      frame "4461: RESET" {
        n332 = Unbundle By Name(w670) -> ("AI task"=w662:refnum<k21>[], "AO task"=w669:refnum<k21>[])
        n333 = local read "simulate?"() -> (w660:bool)
        n334 = call-poly <userlib>:"Empty Array__ogtk.vi"("Array"=w662) -> ("Empty Array?"=w661:bool)  [unwired: 8 in]
        n335 = Or(x=w660, y=w661) -> (x .or. y?=w659:bool)
        n336 = case shown="False" w659 {
          tunnel: w669 -> [w674 _]
          tunnel: w665 -> [w673 w702]
          tunnel: [w672 w702] -> w664
          tunnel: w662 -> [w671 _]
          frame False {
            n337 = disable-structure shown="Default" {
              disable-tunnel: w674 -> [w676 _]
              disable-tunnel: w673 -> [w677 _]
              disable-tunnel: [w678 _] -> w672
              disable-tunnel: w671 -> [w675 _]
              frame condition #0 (active) {
                n338 = for {
                  tunnel: w676 -> [w701] mode=indexing
                  tunnel: [w699] -> w683 mode=indexing
                  tunnel: w677 -> [w698]
                  tunnel: [w697] -> w680
                  n339 = call <vilib>:"DAQmx Stop Task.vi"("task/channels in"=w701, "error in"=w698) -> ("task out"=w699:refnum<k21>, "error out"=w697:errorcluster)  [unwired: 12 in]
                  n340 = Wait (ms)(milliseconds to wait=u32 50) -> ()  [unwired: 1 out]
                }
                n341 = for {
                  tunnel: w675 -> [w696] mode=indexing
                  tunnel: [w694] -> w679 mode=indexing
                  tunnel: w680 -> [w693]
                  tunnel: [w692] -> w682
                  n342 = call <vilib>:"DAQmx Stop Task.vi"("task/channels in"=w696, "error in"=w693) -> ("task out"=w694:refnum<k21>, "error out"=w692:errorcluster)  [unwired: 12 in]
                  n343 = Wait (ms)(milliseconds to wait=u32 50) -> ()  [unwired: 1 out]
                }
                n344 = for {
                  tunnel: w683 -> [w691] mode=indexing
                  tunnel: w682 -> [w689]
                  tunnel: [w688] -> w681
                  n345 = call <vilib>:"DAQmx Clear Task.vi"("task in"=w691, "error in"=w689) -> ("error out"=w688:errorcluster)  [unwired: 13 in]
                  n346 = Wait (ms)(milliseconds to wait=u32 50) -> ()  [unwired: 1 out]
                }
                n347 = for {
                  tunnel: w679 -> [w687] mode=indexing
                  tunnel: w681 -> [w685]
                  tunnel: [w684] -> w678
                  n348 = call <vilib>:"DAQmx Clear Task.vi"("task in"=w687, "error in"=w685) -> ("error out"=w684:errorcluster)  [unwired: 13 in]
                  n349 = Wait (ms)(milliseconds to wait=u32 50) -> ()  [unwired: 1 out]
                }
              }
              frame condition #1 {
              }
            }
          }
          frame True {
          }
        }
        n350 = local write "RESET"(FALSE ("EXIT")) -> ()
        n351 = call <vilib>:"Add State(s) to Queue__JKI_lib_State_Machine.vi"("State(s) in Front (\"\")"="4461: SETUP", "State(s) in (\"\")"=w668) -> ("States Out"=w666:string)  [unwired: 13 in]
      }
      frame "4461: EXIT" {
        n352 = Unbundle By Name(w710) -> ("AO task"=w706:refnum<k21>[], "AI task"=w707:refnum<k21>[])
        n353 = local read "simulate?"() -> (w704:bool)
        n354 = call-poly <userlib>:"Empty Array__ogtk.vi"("Array"=w706) -> ("Empty Array?"=w705:bool)  [unwired: 8 in]
        n355 = Or(x=w704, y=w705) -> (x .or. y?=w703:bool)
        n356 = case shown="False" w703 {
          tunnel: w706 -> [w718 _]
          tunnel: w709 -> [w717 w746]
          tunnel: [w716 w746] -> w708
          tunnel: w707 -> [w715 _]
          frame False {
            n357 = disable-structure shown="Default" {
              disable-tunnel: w718 -> [w726 _]
              disable-tunnel: w717 -> [w725 _]
              disable-tunnel: [w722 _] -> w716
              disable-tunnel: w715 -> [w719 _]
              frame condition #0 (active) {
                n358 = for {
                  tunnel: w719 -> [w745] mode=indexing
                  tunnel: [w743] -> w727 mode=indexing
                  tunnel: w725 -> [w742]
                  tunnel: [w741] -> w721
                  n359 = call <vilib>:"DAQmx Stop Task.vi"("task/channels in"=w745, "error in"=w742) -> ("task out"=w743:refnum<k21>, "error out"=w741:errorcluster)  [unwired: 12 in]
                  n360 = Wait (ms)(milliseconds to wait=u32 50) -> ()  [unwired: 1 out]
                }
                n361 = for {
                  tunnel: w726 -> [w740] mode=indexing
                  tunnel: [w738] -> w720 mode=indexing
                  tunnel: w721 -> [w737]
                  tunnel: [w736] -> w724
                  n362 = call <vilib>:"DAQmx Stop Task.vi"("task/channels in"=w740, "error in"=w737) -> ("task out"=w738:refnum<k21>, "error out"=w736:errorcluster)  [unwired: 12 in]
                  n363 = Wait (ms)(milliseconds to wait=u32 50) -> ()  [unwired: 1 out]
                }
                n364 = for {
                  tunnel: w727 -> [w735] mode=indexing
                  tunnel: w724 -> [w733]
                  tunnel: [w732] -> w723
                  n365 = call <vilib>:"DAQmx Clear Task.vi"("task in"=w735, "error in"=w733) -> ("error out"=w732:errorcluster)  [unwired: 13 in]
                  n366 = Wait (ms)(milliseconds to wait=u32 50) -> ()  [unwired: 1 out]
                }
                n367 = for {
                  tunnel: w720 -> [w731] mode=indexing
                  tunnel: w723 -> [w729]
                  tunnel: [w728] -> w722
                  n368 = call <vilib>:"DAQmx Clear Task.vi"("task in"=w731, "error in"=w729) -> ("error out"=w728:errorcluster)  [unwired: 13 in]
                  n369 = Wait (ms)(milliseconds to wait=u32 50) -> ()  [unwired: 1 out]
                }
              }
              frame condition #1 {
              }
            }
          }
          frame True {
          }
        }
        n370 = Initialize Array(w713, 8 ("dimension size")) -> (w711:i32[])
        n371 = local write "phase log"(w711) -> ()
      }
    }
  }
